vi "DAISY_HIGHSPEED_slow_control_2_16.vi"() -> ()   [LabVIEW 2018]
uses:
  4623b864-5764-45c6-9cb2-3e18237880ca.vi
  fa57f61f-0bb9-49ac-92eb-fcb40add4dbb.vi
  <vilib>/DAQmx/read.llb/DAQmx Read (Analog 1D DBL NChan 1Samp).vi
  ffb0d1b3-ef19-4e2e-b36e-7277177ef4b3.vi
  9a1acc8a-69db-4048-9e4c-bb07d66d2422.vi
  <vilib>/DAQmx/create/channels.llb/DAQmx Create Channel (AI-Voltage-Basic).vi
  <vilib>/DAQmx/create/channels.llb/DAQmx Create Channel (AI-Current-Basic).vi
  <vilib>/DAQmx/create/channels.llb/DAQmx Create Channel (AI-Temperature-RTD).vi
  <vilib>/DAQmx/miscellaneous.llb/DAQmx Fill In Error Info.vi
  <vilib>/Utility/file.llb/Read Delimited Spreadsheet (string).vi
  <instrlib>/Lake Shore 335/Lake Shore 335.lvlib
  <instrlib>/CAEN PSM/CAEN PSM.lvlib
  <resource>/objmgr/daqmx.rc
panel:
  out "Heater":dbl
  out "Coldhead":dbl
  out "Cycle number":i32
  out "Alarm state":bool
  out "Timestamp last \nmeasured (UPS)":timestamp
  out "Auto-clear":bool
  in  "Auto-clear data?":bool
  in  "Clear data":bool
  in  "Clear data every N cycles":dbl=1000000.0
  in  "N samples":i32=30
  out "Average Flow (SLPM)":dbl caption="Flow (SLPM)"
  out "CAEN Ch. Names":string[](array[string])
  in  "Cycles to execute":dbl=5.0 format="%#_13g"
  out "Detector Pressure":dbl
  in  "N samples":i32=20
  in  "Allows tabs on \nfront panel":T1(tab)
  in  "Anode ch.":enum16{"1", "2", "3", "4"}(ring)=enum."3"
  in  "CAEN unit selector":enum16{"CAEN 1", "CAEN 2"}(ring)
  in  "Multipliers":dbl[](array[numeric])=[1.0, 1.0, 1.0, 1.0, 1.0, 1.0, 1.0, 1.0]
  in  "Offsets\nsubtracted":dbl[](array[numeric])=[0.0, 0.0, 0.0, 0.0, 0.0, 0.0, 0.0, 0.0]
  in  "Channel Names (9207, ai8:15)":string[](array[string])=["i0", "i1", "i2", "i3", "i4", "i5", "i6", "i7"] caption="\"Other\""
  in  "Flow meter input:":u16(ring)=3 items=["v0", "v1", "v2", "v3", "v4", "v5", "v6", "v7"]
  in  "Detector pressure input:":u16(ring) items=["v0", "v1", "v2", "v3", "v4", "v5", "v6", "v7"]
  in  "Channel Names (9207, ai0:7)":string[](array[string])=["v0", "v1", "v2", "v3", "v4", "v5", "v6", "v7"] caption="\"Other\""
  in  "Multipliers":dbl[](array[numeric])=[1.0, 1.0, 1.0, 1.0, 1.0, 1.0, 1.0, 1.0]
  in  "Offsets\nsubtracted":dbl[](array[numeric])=[0.0, 0.0, 0.0, 0.0, 0.0, 0.0, 0.0, 0.0]
  in  "Voltage channels":tag[](array[tag])=["9207/ai0", "9207/ai1", "9207/ai2", "9207/ai3", "9207/ai4", "9207/ai5", "9207/ai6", "9207/ai7"]
  in  "COM-port CAEN":refnum<visa-resource-name>
  in  "ID Query":bool
  in  "COM-port LakeShore":refnum<visa-resource-name>
  in  "PID settings":cluster{"P":dbl, "I":dbl, "D":dbl}={"P"=50.0, "I"=20.0, "D"=120.0}
  in  "Current channels":tag[](array[tag])=["9207/ai8", "9207/ai9", "9207/ai10", "9207/ai11", "9207/ai12", "9207/ai13", "9207/ai14", "9207/ai15"]
  in  "Channel Names (CAEN)":string[](array[string])=["PMT 1", "PMT 2", "Anode", "Cathode", "Top gate", "Bottom gate", "Other 1", "Other 2"]
  in  "RTD Type":i32(ring)=10071 items=["Pt3750"=12481, "Pt3851"=10071, "Pt3911"=12482, "Pt3916"=10069, "Pt3920"=10053, "Pt3928"=12483, "Custom"=10137]
  in  "Module 1 channels (slot 1)":tag[](array[tag])=["cDAQ2Mod2/ai0", "cDAQ2Mod2/ai1", "cDAQ2Mod2/ai2", "cDAQ2Mod2/ai3", "cDAQ2Mod2/ai4", "cDAQ2Mod2/ai5", "cDAQ2Mod2/ai6", "cDAQ2Mod2/ai7"]
  in  "Resistance Configuration":i32(ring)=3 items=["3-Wire"=3, "4-Wire"=4]
  in  "R (T = 0°C):":dbl=100.0 format="%_4g"
  in  "B":dbl
  in  "A":dbl
  in  "C":dbl
  in  "Module 2 channels (slot 2)":tag[](array[tag])=["cDAQ2Mod3/ai0", "cDAQ2Mod3/ai1", "cDAQ2Mod3/ai2", "cDAQ2Mod3/ai3", "cDAQ2Mod3/ai4", "cDAQ2Mod3/ai5", "cDAQ2Mod3/ai6", "cDAQ2Mod3/ai7"]
  in  "Shut off heater \nif Alarm is active":bool=TRUE
  in  "Re-save headers":bool
  in  "Resistance Configuration":i32(ring)=3 items=["3-Wire"=3, "4-Wire"=4]
  in  "Module 3 channels":tag[](array[tag])
  in  "RTD Type":i32(ring)=12481 items=["Pt3750"=12481, "Pt3851"=10071, "Pt3911"=12482, "Pt3916"=10069, "Pt3920"=10053, "Pt3928"=12483, "Custom"=10137]
  in  "R (T = 0°C)":dbl=1000.0 format="%0.1f"
  in  "Ignore Initialization Errors":bool=TRUE caption="Ignore init. errors?"
  out "Started up?":bool
  out "heater":i32
  in  "Kill all channels":bool
  in  "Scale.Range:Minimum 8":dbl
  in  "Scale.Range:Maximum 8":dbl=4000.0
  in  "Scale.Range:Minimum 7":dbl
  in  "Scale.Range:Maximum 7":dbl=4000.0
  in  "Scale.Range:Minimum 6":dbl=-3000.0
  in  "Scale.Range:Maximum 6":dbl
  in  "Scale.Range:Minimum 5":dbl
  in  "Scale.Range:Maximum 5":dbl=3000.0
  in  "Scale.Range:Minimum 4":dbl=-5000.0
  in  "Scale.Range:Maximum 4":dbl
  in  "Scale.Range:Maximum 3":dbl=4000.0
  in  "Scale.Range:Minimum 3":dbl
  in  "Scale.Range:Maximum 2":dbl=1000.0
  in  "Scale.Range:Minimum 2":dbl
  out "CAEN 1.1":dbl(knob) scale=0.0..1000.0
  out "CAEN 1.1":string
  in  "Scale.Range:Maximum":dbl=1000.0
  in  "Scale.Range:Minimum":dbl
  out "CAEN 2.3 2":string
  out "CAEN 2.2 2":string
  out "Channel Names":string[](array[string])
  out "CAEN 2.3":dbl(knob) scale=0.0..4000.0
  out "CAEN 2.2":dbl(knob) scale=0.0..4000.0
  out "CAEN 2.1":string
  out "CAEN 2.0":string
  out "CAEN 1.3":string
  out "CAEN 1.2":string
  out "CAEN 1.0":string
  out "Channel Names":string[](array[string])
  in  "Set to zero (ramp down)":bool
  out "CAEN 2.1":dbl(knob) scale=0.0..-3000.0
  out "CAEN 2.0":dbl(knob) scale=0.0..3000.0
  in  "Apply Voltage":bool
  in  "VSet (V)":dbl[](array[numeric])
  in  "IMax (uA)":dbl[](array[numeric])
  in  "VMax (V)":dbl[](array[numeric])
  out "CAEN 1.3":dbl(knob) scale=0.0..-5000.0
  out "CAEN 1.2":dbl(knob) scale=0.0..4000.0
  out "CAEN 1.0":dbl(knob) scale=0.0..1000.0
  out "Vmon (V)":dbl[](array[numeric])
  out "IMon (uA)":dbl[](array[numeric])
  in  "Reset anode\nperiodically?":bool
  in  "Kill every Y minutes":i32=10
  in  "Keep off for X seconds":i32=10
  out "?":bool
  out "Killed":bool
  out "Restarted":bool
  out "Anode timers":timestamp[](array[timestamp])
  out "Seconds until \nanode autokill":dbl format="%.2g"
  out "Seconds until \nanode reset":dbl format="%.2g"
  in  "Temperature channel selector":u16(ring) items=["0"=0, "1"=1, "2"=2, "3"=3, "4"=4, "5"=5, "6"=6, "7"=7, "Average"=666]
  out "Heater power (%)":cluster{timestamp[], dbl[]}[](graph)
  out "Flow (SLPM)":cluster{timestamp[], dbl[]}[](graph)
  out "9207 (ai 0:7, Volts)":cluster{timestamp[], dbl[]}[](graph)
  out "Phase Diagram":cluster{"X":dbl, "Y":dbl}[](graph)
  out "Setup Temperature (9216 0:15, °C)":cluster{timestamp[], dbl[]}[](graph)
  out "LakeShore readings":dbl[](array[numeric])
  out "Low Temperature (9226 0:7 and LakeShore A;B, °C)":cluster{timestamp[], dbl[]}[](graph)
  in  "Reset?":bool
  out "Integrated Flow (SL)":dbl
  in  "Pause?":bool
  in  "Setpoint (°C)":dbl=-100.0 format="%.1f"
  in  "Heater range":u16(ring) items=["Off", "Low (On)", "Medium", "High"]
  in  "\"Sound\" alarm":bool
  in  "Sound alarm\nFrequency (Hz)":dbl=1260.0
  in  "Send status email now":bool
  out "Email error":i32
  out "source":string
  in  "Number of Bonus lines":i32=1
  out "Names (optional)":string[](array[string])
  in  "Send daily email?":bool=TRUE
  in  "Phone numbers":string[](array[string])
  out "Alarm (or test) message":string
  in  "Alarm\nMaster switch":bool
  in  "Repeat Alarm SMS\nevery N minutes":dbl=15.0
  in  "Test alarm":bool
  out "Warning":bool
  in  "UPS":bool
  in  "UPS Voltage \nLower Threshold":dbl=220.0
  out "NI mod 2&3 status":bool
  in  "NI mod 2&3":bool
  in  "NI mod 1":bool
  in  "CAEN 2":bool
  in  "CAEN 1":bool
  in  "LakeShore":bool
  out "Det. P. warning":bool
  out "Boolean 6":bool
  out "Boolean 5":bool
  out "Boolean 4":bool
  out "Boolean 3":bool
  out "Boolean 2":bool
  out "Boolean":bool
  in  "T 6":bool
  in  "T 5":bool
  in  "T 4":bool
  in  "T 3":bool
  in  "T 2":bool
  in  "T 1":bool
  in  "Detector Pressure":bool
  in  "Overpressure threshold":dbl
  in  "Underpressure threshold":dbl
  out "Comm. status":bool
  in  "High Temp threshold":dbl format="%#_13g"
  in  "Low Temp threshold":dbl format="%#_13g"
  out "LakeShore status":bool
  out "NI mod1 (P) status":bool
  out "CAEN 1 status":bool
  out "CAEN 2 status":bool
  out "Initialization status":bool
  out "Minimum input voltage measured":dbl
  out "Alarm active 2":bool
  out "SMS error":string
  out "Status email preview":string
  in  "Send status email at time:":string="14:00"
  in  "Email Addresses":string[](array[string])
  in  "return address":string="xamsups@gmail.com"
  out "NI 9226":errorcluster
  in  "HV Channel status":string="Click the button to request the latest High Voltage channel status.\nView another channel with the arrows, or typing 0 through 3."
  out "CAEN 1":T2(array[cluster])
  out "CAEN 2":T2(array[cluster])
  in  "Query HV status":bool
  in  "LabVIEW error code":string="Google this"
  in  "String 7":string="A checkmark means \"No error\" and false. A red X means an error occurred"
  out "\"status\"":bool
  in  "\"source\"":string="This may show two things: the latest executed VI in the task chain, in reverse order, or: which VI produced an error, with a short description. If the error can't easily be resolved, google the code."
  out "NI 9216 x2":errorcluster
  out "CAEN 1":errorcluster
  out "CAEN 2":errorcluster
  out "Lakeshore":errorcluster
  out "NI 9207":errorcluster
  out "Temp A":dbl
  out "Temp B":dbl
  in  "Temperature Channel Selector":u16(ring) items=["0", "1", "2", "3", "4", "5", "6", "7"]
  out "Historical Large Phase Diagram":cluster{dbl[], dbl[]}[](graph)
  out "Large Phase Diagram":cluster{"X":dbl, "Y":dbl}[](graph)
  in  "Temperature Channel Selector":u16(ring) items=["0"=0, "1"=1, "2"=2, "3"=3, "4"=4, "5"=5, "6"=6, "7"=7, "Average"=666]
  out "PT1000 data":dbl[](array[numeric]) format="%0.2f"
  out "9207 (V; A) Converted":dbl[](array[numeric])
  out "9216 #1 (°C)":dbl[](array[numeric])
  out "9216 #2 (°C)":dbl[](array[numeric])
  out "Raw readouts (V, mA)":dbl[](array[numeric]) format="%0.2f"
  out "Det.P input #":i32
  out "Flow input #":i32
  out "PT100 data":dbl[](array[numeric]) format="%0.2f"
  out "9207 (ai 8:15, Amperes)":cluster{timestamp[], dbl[]}[](graph)
  in  "Kill voltage":bool
  in  "stop":bool
  out "Voltages":dbl[](array[numeric])
  out "TOBA appended":dbl[][](array[numeric])
  out "Time until next cycle":dbl format="%.3g"
  in  "Time per cycle (s)":i32=2 caption="Time Target (s)"
  # "<- Proof of concept for New/Old T + New P"
  # "Remove ^this^ array, just for testing and takes up lots of resources"
  # "Moving averages"
  # "CAEN settings"
  # "NI 9216 Temperature settings"
  # "NI 9207 Voltage settings"
  # "NI 9207 Current settings"
  # "If RTD type is custom,\nspecify the Callendar-\nVan Dusen parameters"
  # "Anode connected to:"
  # "Channel:"
  # "Lakeshore settings"
  # "NI 9226 Temperature settings"
  # "Miscellaneous"
  # "Gain (P) (XX.X)"
  # "Reset (I) (XX.X)"
  # "Rate (D) (X.X%)"
  # "Data"
  # "Scale:"
  # "to"
  # "to"
  # "Scale:"
  # "Time of last reset"
  # "Time of last reactivation"
  # "to"
  # "Scale:"
  # "to"
  # "Scale:"
  # "Settings"
  # "Scale:"
  # "to"
  # "Scale:"
  # "to"
  # "Scale:"
  # "to"
  # "to"
  # "Scale:"
  # "Alarm indicators and arms"
  # "Detector Thresholds"
  # "Daily status email"
  # "SMS and sound alarm"
  # "Alarm conditions"
  # "Temperature channels:"
  # "Uninterruptable Power Supply"
  # "Task information"
  # "High Voltage channel status"
  # "Error info example"
  # "Channel"
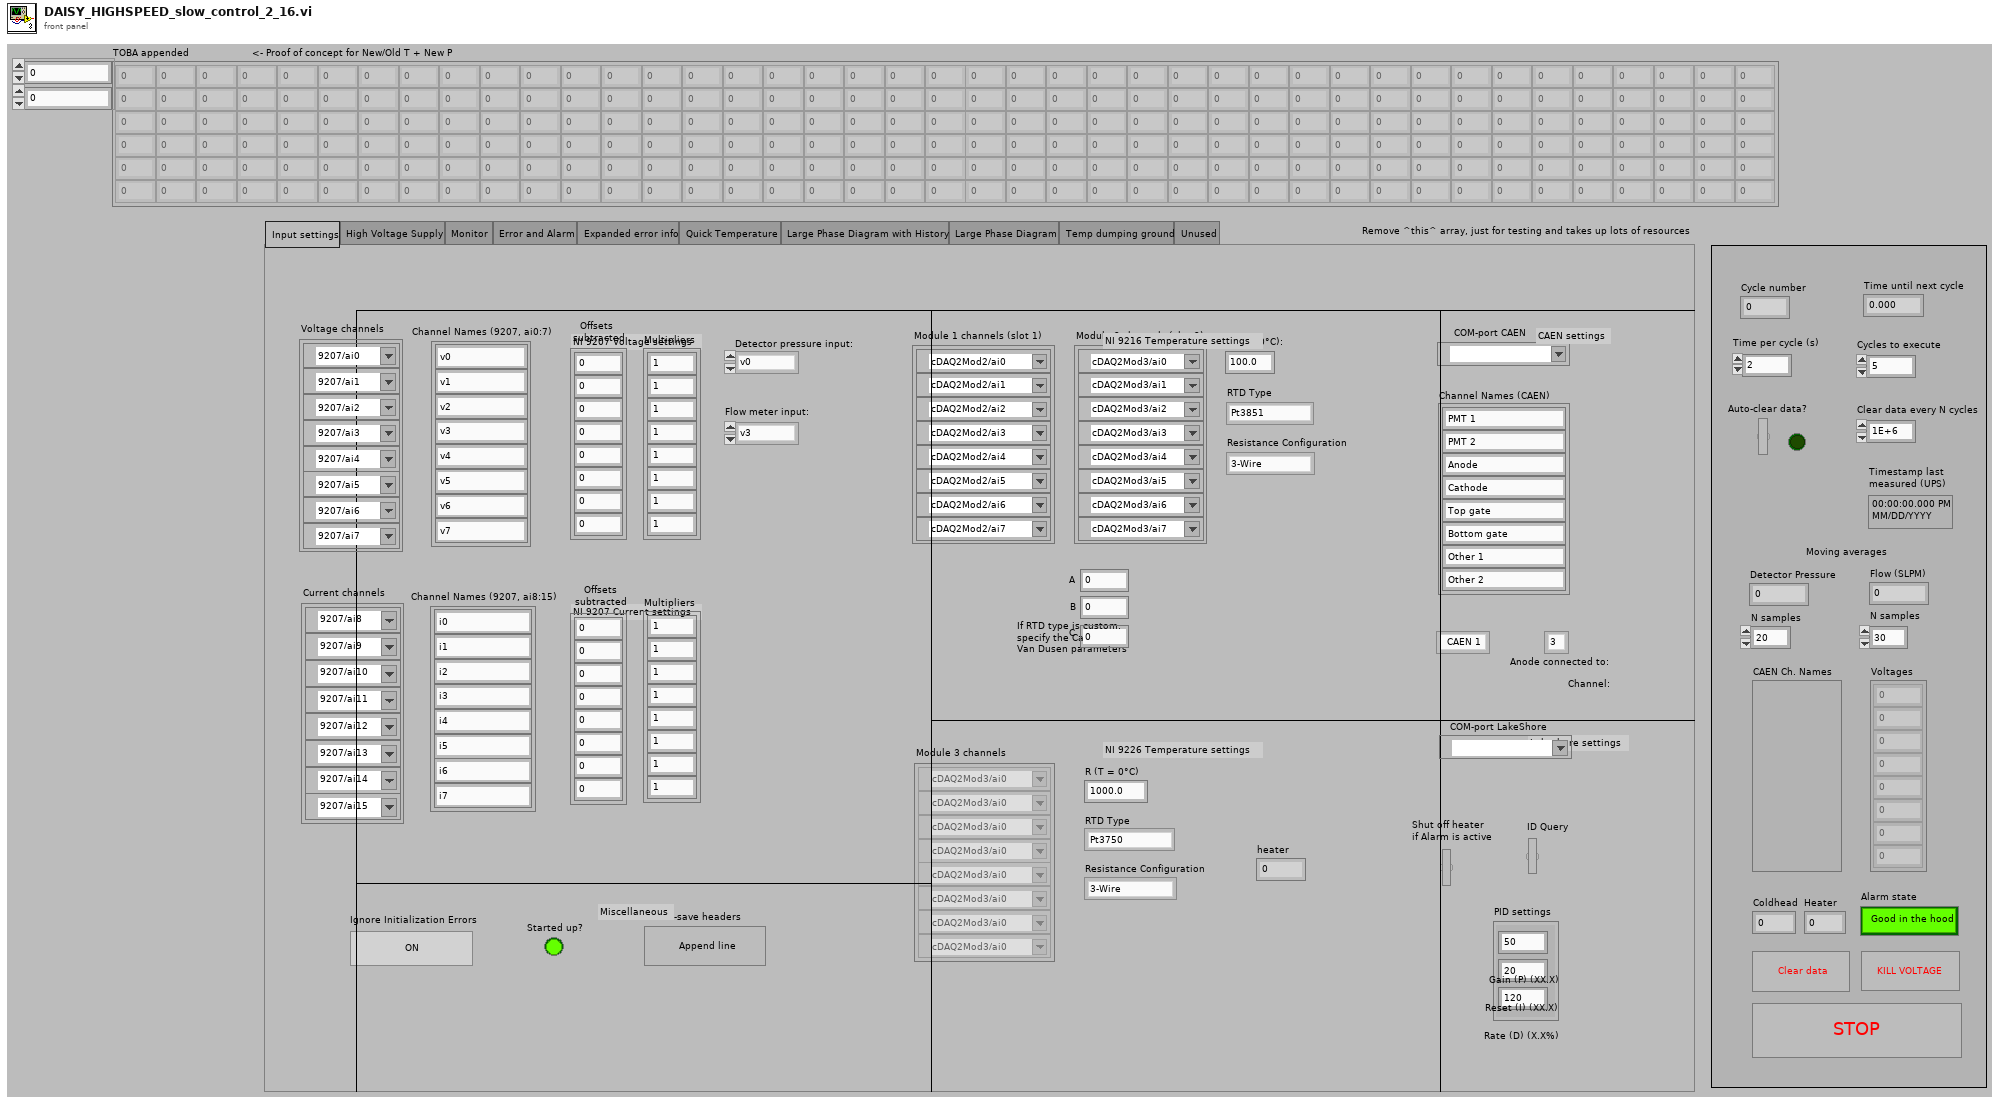
[diagram p1: front panel]
types:
  T1 = enum32{"Input settings", "High Voltage Supply", "Monitor", "Error and Alarm", "Expanded error info", "Quick Temperature", "Large Phase Diagram with History", "Large Phase Diagram", "Temp dumping ground", "Unused"}
  T2 = cluster{"ON":bool, "RUP":bool, "RDW":bool, "OVC":bool, "OVV":bool, "UNV":bool, "MAXV":bool, "TRIP":bool, "OVP":bool, "OVT":bool, "DIS":bool, "KILL":bool, "ILK":bool, "NOCAL":bool}[]
  T3 = cluster{"Baud Rate":u32, "Parity":u16, "Data Bits":u16, "Stop Bits":u16, "Flow Control":u16}
  T4 = typedef "CAEN PSM.lvlib/BoardHandle.ctl" = cluster{"VISA resource name":refnum<visa-resource-name>, "Board address":u8, "NChannels":u8}
  T5 = cluster{"task out":refnum<k21>, "error out":errorcluster}
  T6 = cluster{"VISA resource name out":refnum<visa-resource-name>, "error out":errorcluster}
  T7 = cluster{"VISA resource name":refnum<visa-resource-name>, "Board address":u8, "NChannels":u8}[]
  T8 = cluster{"VISA resource name":refnum<visa-resource-name>, "Board address":u8, "NChannels":u8}
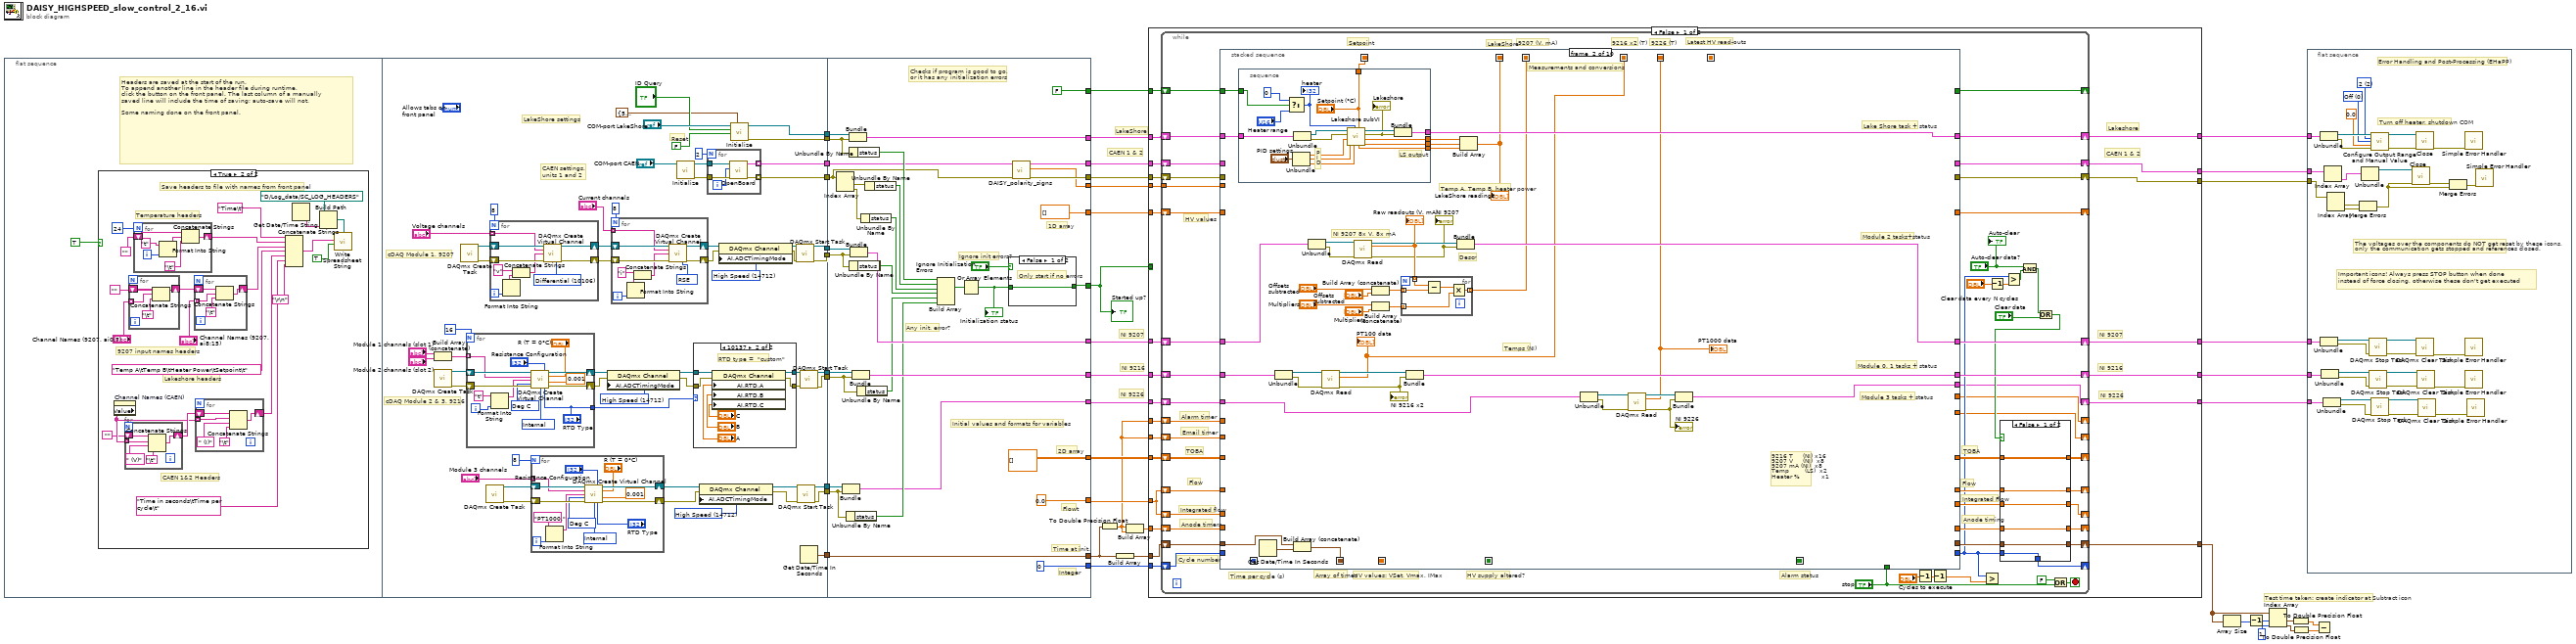
[diagram p0: block diagram]
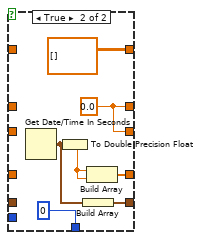
[diagram p2: hidden frame]
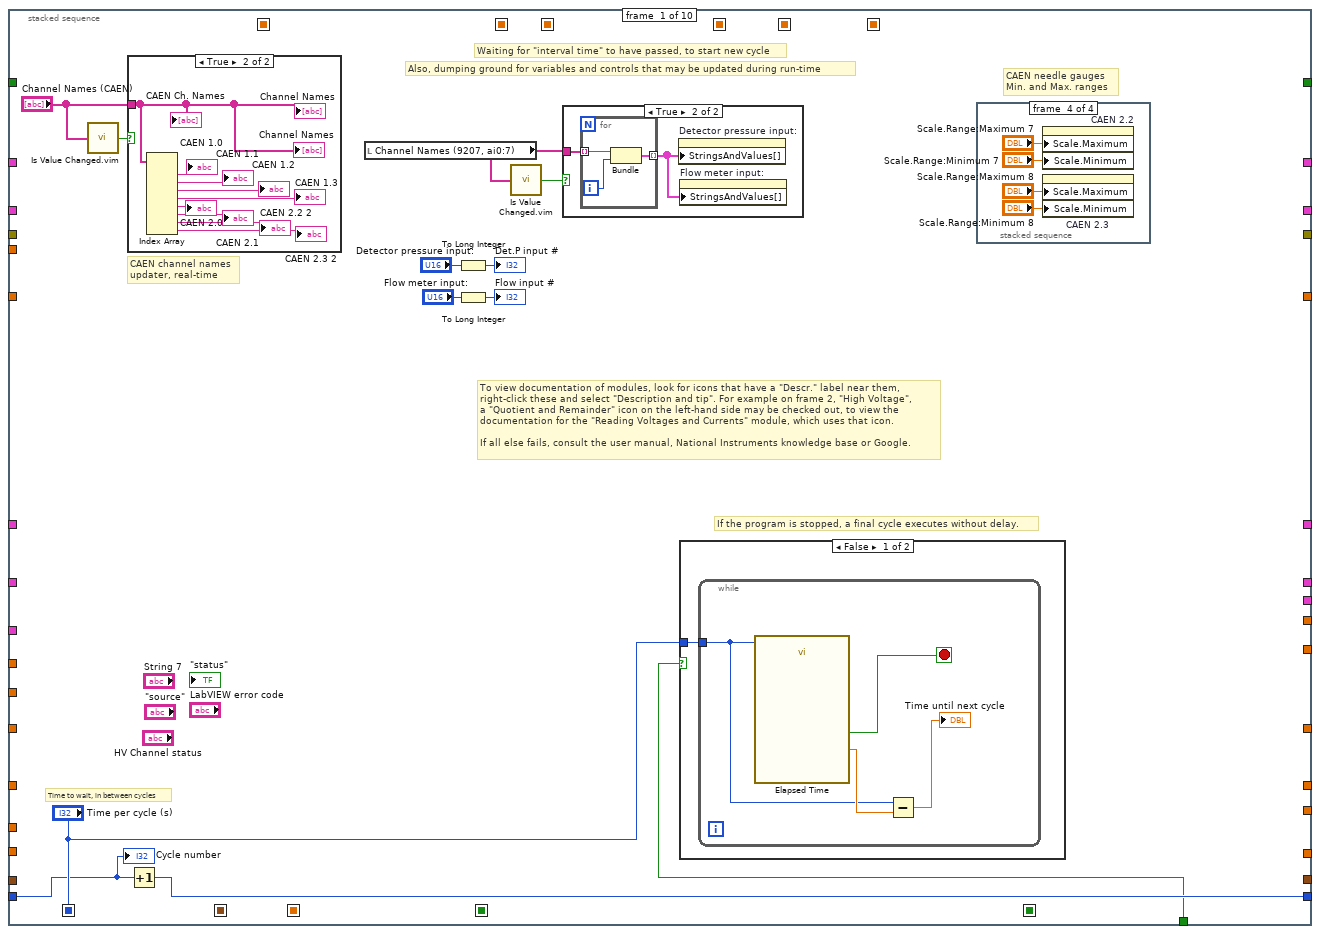
[diagram p3: hidden frame]
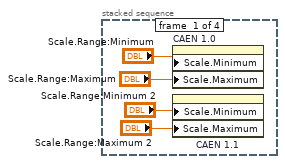
[diagram p6: hidden frame]
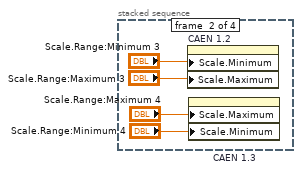
[diagram p7: hidden frame]
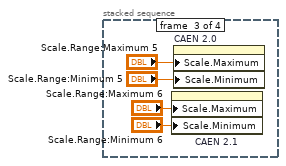
[diagram p8: hidden frame]
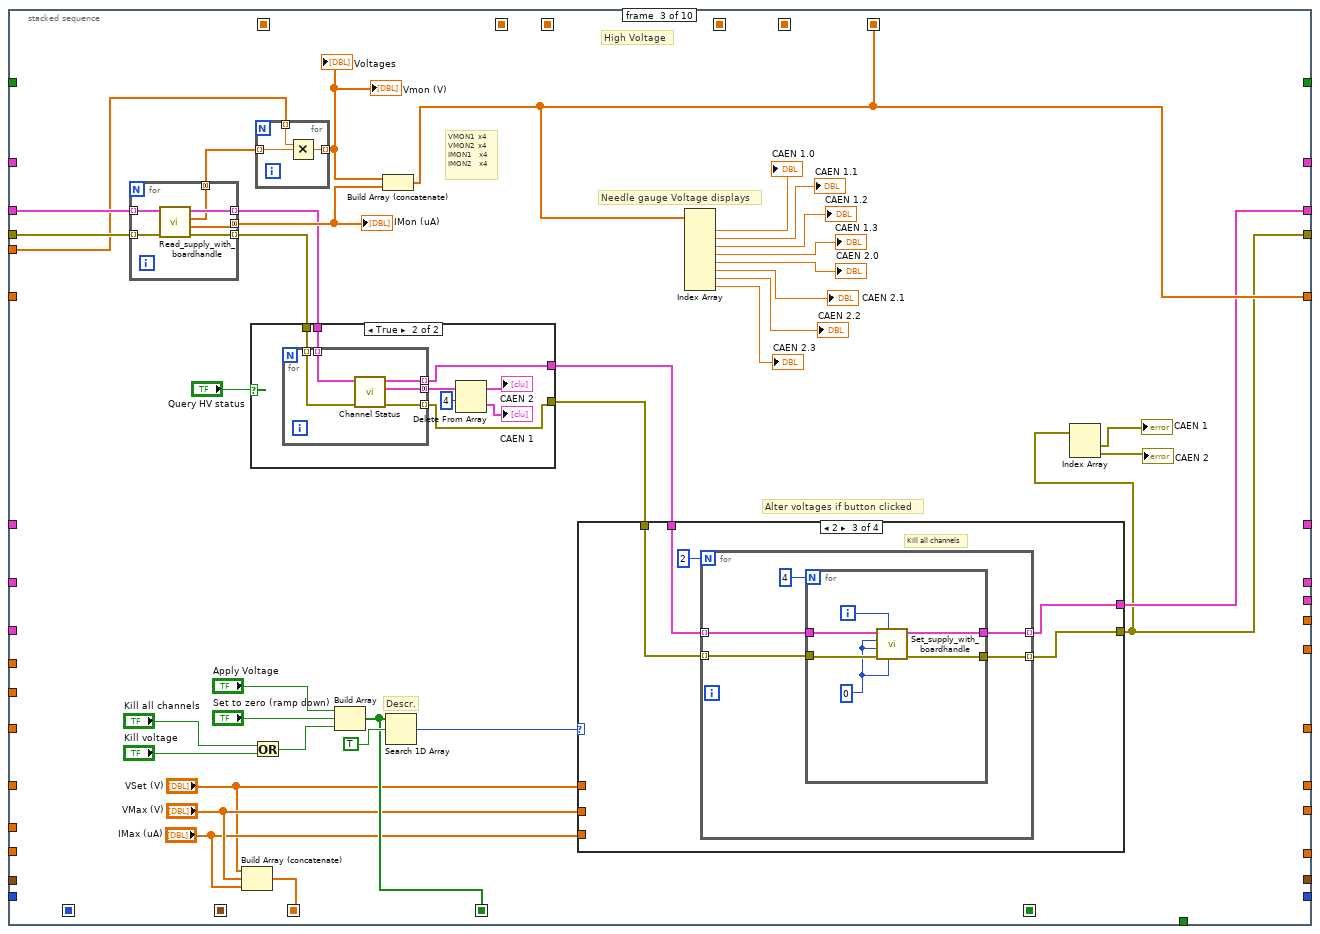
[diagram p10: hidden frame]
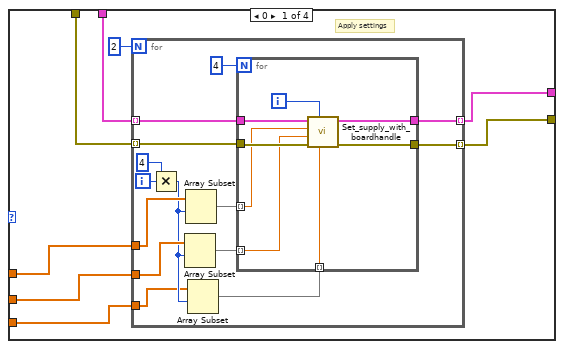
[diagram p11: hidden frame]
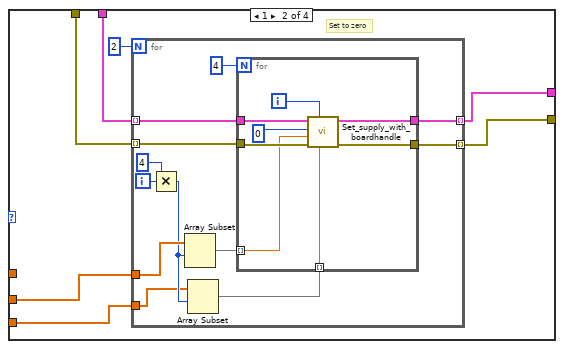
[diagram p12: hidden frame]
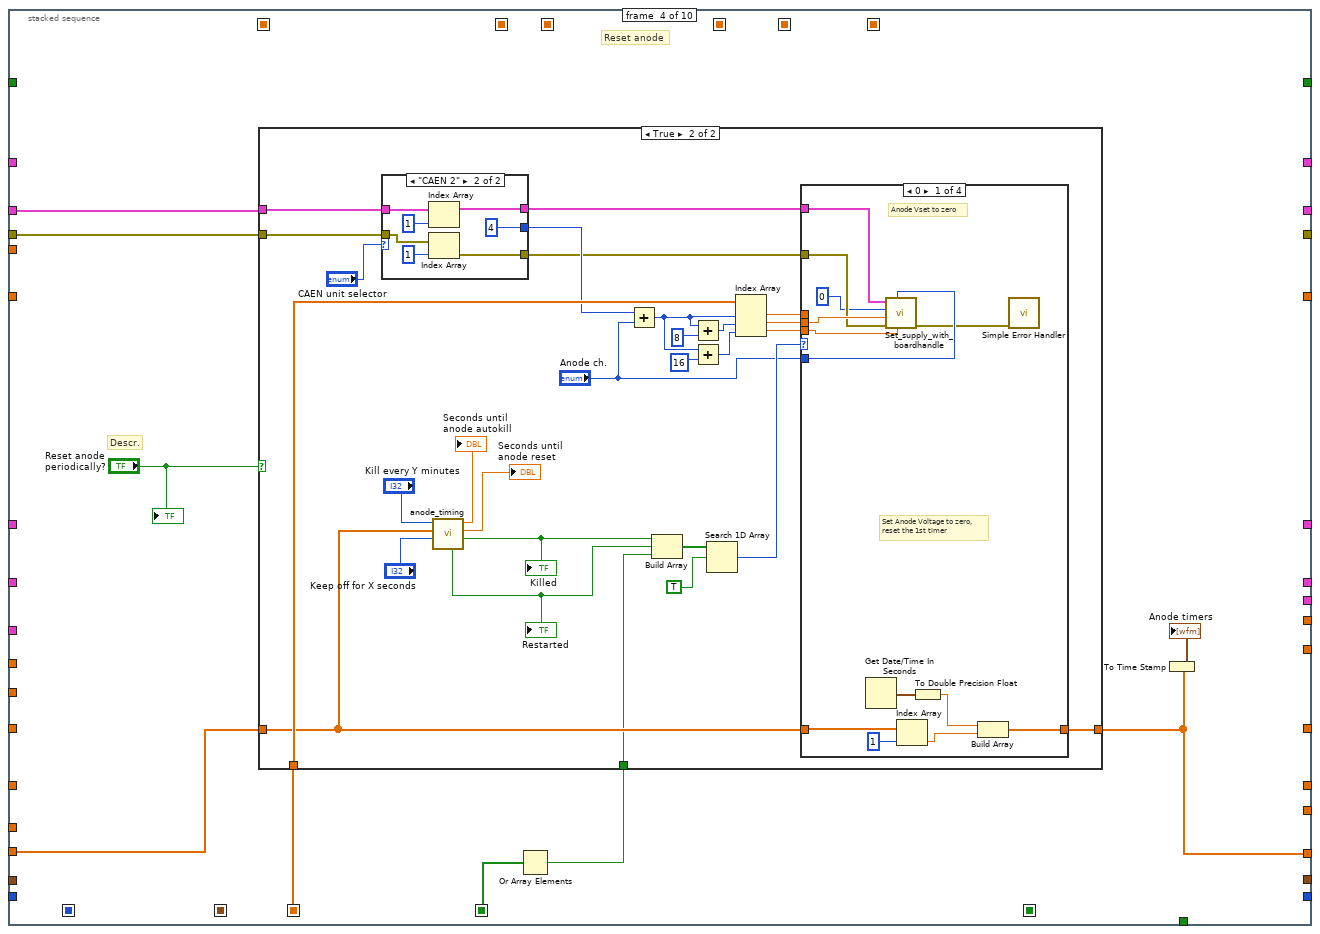
[diagram p15: hidden frame]
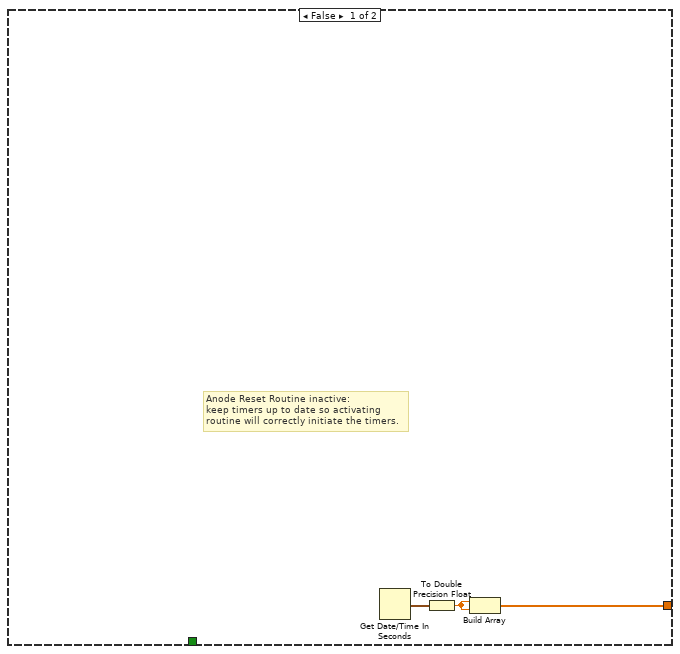
[diagram p16: hidden frame]
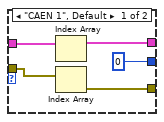
[diagram p17: hidden frame]
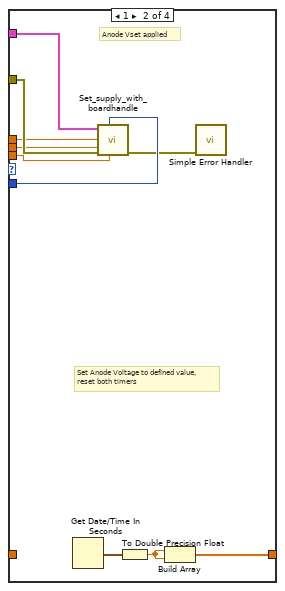
[diagram p18: hidden frame]
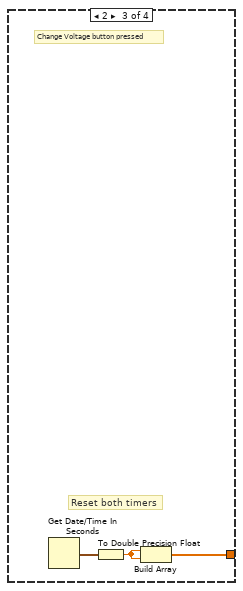
[diagram p19: hidden frame]
diagram:
  # "NI 9226"
  # "NI 9216"
  # "Test time taken: create indicator at Subtract icon"
  # "NI 9207"
  # "CAEN 1 & 2"
  # "LakeShore"
  n1 = flat-sequence {
    tunnel: [w140] -> w42
    tunnel: [w139] -> w41
    tunnel: [w136] -> w40
    tunnel: [w127] -> w39
    tunnel: [w135] -> w35
    tunnel: [w128] -> w21
    tunnel: [w122] -> w14
    tunnel: [w121] -> w13
    tunnel: [w110] -> w9
    tunnel: [w109] -> w8
    tunnel: [w106] -> w4
    tunnel: w42 -> [w237]
    tunnel: w41 -> [w236]
    tunnel: w40 -> [w208]
    tunnel: w39 -> [w229]
    tunnel: [w238] -> w27
    tunnel: [0.0] -> w26
    tunnel: [dbl[] []] -> w38
    tunnel: [dbl[][] []] -> w15
    tunnel: [0] -> w37
    tunnel: [w235] -> w36
    tunnel: [w234] -> w25
    tunnel: w35 -> [w234]
    tunnel: [FALSE] -> w22
    tunnel: w21 -> [w230]
    tunnel: [w228] -> w20
    tunnel: w14 -> [w221]
    tunnel: w13 -> [w220]
    tunnel: [w219] -> w12
    tunnel: w9 -> [w216]
    tunnel: w8 -> [w215]
    tunnel: [w213] -> w7
    tunnel: [w206] -> w5
    tunnel: w4 -> [w210]
    tunnel: [w209] -> w3
    tunnel: [w207] -> w2
    frame #0 {
      # "Headers are saved at the start of the run.\nTo append another line in the header file during runtime,\nclick the button on the front panel. The last column of a manually\nsaved line will include the time of saving; auto-save will not.\n\nSome naming done on the front panel."
      n2 = case shown="True" TRUE {
        frame False {
        }
        frame True {
          # "CAEN 1&2 Headers"
          # "Lakeshore headers"
          # "9207 input names headers"
          # "Temperature headers"
          # "Save headers to file with names from front panel"
          n3 = property on="Channel Names (CAEN)" class="Arr (strict)"() -> ("Value"=w49:string[])  [unwired: 2 in, 2 out]
          n4 = for {
            tunnel: w49 -> [w73] mode=indexing
            shift-right: [w71] -> w50
            shift-left: "" -> [w70]
            n5 = Concatenate Strings(w70, w73, " (V)", "\t") -> (w71:string)
          }
          n6 = for {
            shift-right: [w81] -> w53
            shift-left: "" -> [w82]
            tunnel: "Channel Names (9207, ai0:7)" -> [w79] mode=indexing
            n7 = Concatenate Strings(w82, w79, "\t") -> (w81:string)
          }
          n8 = for {
            N: 24 -> [_]
            shift-right: [w83] -> w56
            shift-left: "" -> [w84]
            i -> [w88]
            n9 = Format Into String(initial string="t", w88) -> (resulting string=w86:string)  [unwired: 2 in, 1 out]
            n10 = Concatenate Strings(w84, w86, "\t") -> (w83:string)
          }
          n11 = for {
            shift-right: [w76] -> w52
            shift-left: w53 -> [w78]
            tunnel: "Channel Names (9207, ai8:15)" -> [w75] mode=indexing
            n12 = Concatenate Strings(w78, w75, "\t") -> (w76:string)
          }
          n13 = for {
            shift-right: [w66] -> w48
            shift-left: w50 -> [w67]
            tunnel: w49 -> [w65] mode=indexing
            n14 = Concatenate Strings(w67, w65, " (I)", "\t") -> (w66:string)
          }
          n15 = Concatenate Strings("Time\t", w56, w52, "Temp A\tTemp B\tHeater Power\tSetpoint\t", w48, "Time in seconds\tTime per cycle\t", "\r\n") -> (w55:string)
          n16 = Get Date/Time String() -> (date string=w59:string)  [unwired: 3 in, 1 out]
          n17 = Build Path(base path=path "D:/Log_data/SC_LOG_HEADERS" ("file path (dialog if empty)"), name or relative path=w59) -> (appended path=w60:path)
          n18 = call <vilib>:"Write Spreadsheet String.vi"("append to file? (new file:F)"=TRUE, "spreadsheet string"=w55, "file path (dialog if empty)"=w60) -> ()  [unwired: 7 in, 2 out]
        }
      }
    }
    frame #1 {
      w89 = 14712 items=["Automatic"=16097, "High Resolution"=10195, "High Speed"=14712, "Best 50 Hz Rejection"=14713, "Best 60 Hz Rejection"=14714, "Custom"=10137] ("AI.ADCTimingMode")
      w94 = 14712 items=["Automatic"=16097, "High Resolution"=10195, "High Speed"=14712, "Best 50 Hz Rejection"=14713, "Best 60 Hz Rejection"=14714, "Custom"=10137] ("AI.ADCTimingMode")
      w101 = 14712 items=["Automatic"=16097, "High Resolution"=10195, "High Speed"=14712, "Best 50 Hz Rejection"=14713, "Best 60 Hz Rejection"=14714, "Custom"=10137] ("AI.ADCTimingMode")
      # "cDAQ Module 2 & 3, 9216"
      # "cDAQ Module 1, 9207"
      # "CAEN settings,\nunits 1 and 2"
      # "Reset"
      # "LakeShore settings"
      n19 = call <vilib>:"DAQmx Create Task.vi"() -> ("task out"=w107:refnum<k21>, "error out"=w123:errorcluster)  [unwired: 14 in]
      n20 = Build Array (concatenate)("Module 1 channels (slot 1)", "Module 2 channels (slot 2)") -> (w118:tag[])
      n21 = call <vilib>:"DAQmx Create Task.vi"() -> ("task out"=w132:refnum<k21>, "error out"=w131:errorcluster)  [unwired: 14 in]
      n22 = for {
        N: 16 -> [_]
        shift-right: [w182] -> w98
        shift-left: w107 -> [w185]
        shift-right: [w183] -> w96
        shift-left: w123 -> [w184]
        tunnel: w118 -> [w181] mode=indexing
        tunnel: ["RTD Type"] -> w115
        i -> [w179]
        w177 = 10200 items=["Internal"=10200, "External"=10167, "None"=10230] ("Current Excitation Source")
        w176 = 10143 items=["Deg C"=10143, "Deg F"=10144, "Kelvins"=10325, "Deg R"=10145, "From Custom Scale"=10065] ("units")
        n23 = Format Into String(initial string="t", w179) -> (resulting string=w178:string)  [unwired: 2 in, 1 out]
        n24 = call-poly <vilib>:"DAQmx Create Virtual Channel.vi"("task in"=w185, "resistance configuration"="Resistance Configuration", "physical channels"=w181, "r0"="R (T = 0°C):", "name to assign"=w178, "units"=w176, "current excitation value"=0.001, "error in"=w184, "current excitation source"=w177, "rtd type"="RTD Type") -> ("task out"=w182:refnum<k21>, "error out"=w183:errorcluster)  [unwired: 4 in]
      }
      n25 = call <vilib>:"DAQmx Create Task.vi"() -> ("task out"=w113:refnum<k21>, "error out"=w112:errorcluster)  [unwired: 14 in]
      n26 = for {
        N: 8 -> [_]
        shift-right: [w201] -> w104
        shift-left: w132 -> [w200]
        shift-right: [w202] -> w129
        shift-left: w131 -> [w198]
        tunnel: "Voltage channels" -> [w199] mode=indexing
        i -> [w204]
        w196 = 10106 items=["Default"=-1, "RSE"=10083, "NRSE"=10078, "Differential"=10106, "Pseudodifferential"=12529] ("input terminal configuration")
        n27 = Format Into String(w204) -> (resulting string=w203:string)  [unwired: 3 in, 1 out]
        n28 = Concatenate Strings("v" ("string"), w203) -> (w197:string)
        n29 = call-poly <vilib>:"DAQmx Create Virtual Channel.vi"("task in"=w200, "input terminal configuration"=w196, "physical channels"=w199, "name to assign"=w197, "error in"=w198) -> ("task out"=w201:refnum<k21>, "error out"=w202:errorcluster)  [unwired: 9 in]
      }
      n30 = for {
        N: 8 -> [_]
        shift-right: [w160] -> w103
        shift-left: w113 -> [w159]
        shift-right: [w161] -> w102
        shift-left: w112 -> [w162]
        tunnel: "Module 3 channels" -> [w157] mode=indexing
        i -> [w155]
        w151 = 10200 items=["Internal"=10200, "External"=10167, "None"=10230] ("current excitation source")
        w153 = 10143 items=["Deg C"=10143, "Deg F"=10144, "Kelvins"=10325, "Deg R"=10145, "From Custom Scale"=10065] ("units")
        n31 = Format Into String(initial string="PT1000.", w155) -> (resulting string=w154:string)  [unwired: 2 in, 1 out]
        n32 = call-poly <vilib>:"DAQmx Create Virtual Channel.vi"("task in"=w159, "resistance configuration"="Resistance Configuration", "physical channels"=w157, "r0"="R (T = 0°C)", "name to assign"=w154, "units"=w153, "current excitation value"=0.001, "error in"=w162, "current excitation source"=w151, "rtd type"="RTD Type") -> ("task out"=w160:refnum<k21>, "error out"=w161:errorcluster)  [unwired: 4 in]
      }
      n33 = property class="DAQmx Channel"(reference=w98, error in=w96, "AI.ADCTimingMode"=w94) -> (reference out=w97:refnum<k21>, error out=w95:errorcluster)
      n34 = for {
        N: 8 -> [_]
        shift-right: [w187] -> w93
        shift-left: w104 -> [w194]
        shift-right: [w186] -> w90
        shift-left: w129 -> [w193]
        tunnel: "Current channels" -> [w192] mode=indexing
        i -> [w191]
        w195 = 10083 items=["default"=-1, "RSE"=10083, "NRSE"=10078, "Differential"=10106, "Pseudodifferential"=12529] ("input terminal configuration")
        n35 = Format Into String(w191) -> (resulting string=w189:string)  [unwired: 3 in, 1 out]
        n36 = Concatenate Strings("i", w189) -> (w188:string)
        n37 = call-poly <vilib>:"DAQmx Create Virtual Channel.vi"("task in"=w194, "input terminal configuration"=w195, "physical channels"=w192, "name to assign"=w188, "error in"=w193) -> ("task out"=w187:refnum<k21>, "error out"=w186:errorcluster)  [unwired: 9 in]
      }
      n38 = call <instrlib>:"Initialize.vi"("VISA resource name"="COM-port CAEN") -> ("error out"=w137:errorcluster, "VISA resource name out"=w133:refnum<visa-resource-name>)  [unwired: 9 in]
      n39 = case shown="10137" w115 {
        tunnel: w97 -> [w164 w168]
        tunnel: w95 -> [w163 w167]
        tunnel: [w164 w166] -> w117
        tunnel: [w163 w165] -> w116
        frame 0, Default {
          # "Don't need to specify the A, B, C\nvalues if RTD type is not \"custom\""
        }
        frame 10137 {
          # "RTD type =  \"custom\""
          n40 = property class="DAQmx Channel"(reference=w168, error in=w167, "AI.RTD.A"="A", "AI.RTD.B"="B", "AI.RTD.C"="C") -> (reference out=w166:refnum<k21>, error out=w165:errorcluster)
        }
      }
      n41 = property class="DAQmx Channel"(reference=w103, error in=w102, "AI.ADCTimingMode"=w101) -> (reference out=w100:refnum<k21>, error out=w99:errorcluster)
      n42 = for {
        N: 2 -> [_]
        tunnel: w133 -> [w146]
        tunnel: [w144] -> w106 mode=indexing
        tunnel: w137 -> [w148]
        tunnel: [w147] -> w136 mode=indexing
        i -> [w145]
        n43 = call <instrlib>:"OpenBoard.vi"("error in (no error)"=w148, "Board Address"=w145, "VISA resource name"=w146) -> ("error out"=w147:errorcluster, "BoardHandle"=w144:T4)  [unwired: 7 in]
      }
      n44 = property class="DAQmx Channel"(reference=w93, error in=w90, "AI.ADCTimingMode"=w89) -> (reference out=w92:refnum<k21>, error out=w91:errorcluster)
      n45 = call <instrlib>:"Initialize.vi"("Serial Configuration"=T3 {"Baud Rate"=57600, "Parity"=1, "Data Bits"=7, "Stop Bits"=10, "Flow Control"=0}, "Reset (True)"=FALSE ("Reset (LakeShore)"), "ID Query (True)"="ID Query", "VISA resource name"="COM-port LakeShore") -> ("error out"=w139:errorcluster, "VISA resource name out"=w140:refnum<visa-resource-name>)  [unwired: 6 in]
      n46 = call <vilib>:"DAQmx Start Task.vi"("task/channels in"=w92, "error in"=w91) -> ("task out"=w128:refnum<k21>, "error out"=w127:errorcluster)  [unwired: 12 in]
      n47 = call <vilib>:"DAQmx Start Task.vi"("task/channels in"=w100, "error in"=w99) -> ("task out"=w110:refnum<k21>, "error out"=w109:errorcluster)  [unwired: 12 in]
      n48 = call <vilib>:"DAQmx Start Task.vi"("task/channels in"=w117, "error in"=w116) -> ("task out"=w122:refnum<k21>, "error out"=w121:errorcluster)  [unwired: 12 in]
      n49 = Get Date/Time In Seconds() -> (seconds since 1Jan1904=w135:timestamp)
    }
    frame #2 {
      # "1D array"
      # "Initial values and formats for variables"
      # "Time at init."
      # "Integer"
      # "2D array"
      # "Flowt"
      # "Checks if program is good to go,\nor it has any initialization errors"
      # "Ignore init errors?"
      # "Any init. error?"
      n50 = Index Array(array=w208) -> (element #1=w212:errorcluster, element #2=w211:errorcluster)  [unwired: 2 in]
      n51 = Bundle("task out"=w216, "error out"=w215) -> (w213:T5)  [unwired: 1 in]
      n52 = Unbundle By Name(w215) -> ("status"=w214:bool)
      n53 = Unbundle By Name(w236) -> ("status"=w222:bool)
      n54 = Bundle("VISA resource name out"=w237, "error out"=w236) -> (w235:T6)  [unwired: 1 in]
      n55 = Unbundle By Name(w229) -> ("status"=w223:bool)
      n56 = Bundle("task out"=w230, "error out"=w229) -> (w228:T5)  [unwired: 1 in]
      n57 = Bundle("task out"=w221, "error out"=w220) -> (w219:T5)  [unwired: 1 in]
      n58 = Unbundle By Name(w220) -> ("status"=w218:bool)
      n59 = Unbundle By Name(w211) -> ("status"=w233:bool)
      n60 = Unbundle By Name(w212) -> ("status"=w239:bool)
      n61 = Build Array(w222, w239, w223, w233, w218, w214) -> (w240:bool[])
      n62 = Or Array Elements(Boolean array=w240) -> (logical OR=w217:bool)
      "Initialization status" <- w217
      n63 = case shown="False" "Ignore Initialization Errors" {
        tunnel: [w241 FALSE] -> w238
        tunnel: w217 -> [w241 _]
        frame False {
          # "Only start if no errors"
        }
        frame True {
          # "Always start program"
        }
      }
      n64 = call "DAISY_polarity_signs.vi"("Errors in"=w208, "BoardHandles"=w210) -> ("Errors out"=w207:errorcluster[], "Polarity signs"=w206:dbl[], "BoardHandles Out"=w209:T7)  [unwired: 7 in]
    }
  }
  n65 = To Double Precision Float(number=w25) -> (double precision float=w10:dbl)
  n66 = Build Array(w25) -> (w34:timestamp[])
  n67 = Build Array(w10, w10) -> (w24:dbl[])
  n68 = case shown="False" w27 {
    selector: w27 -> [_ w1091]
    tunnel: [_ w1091] -> _
    tunnel: w38 -> [w260 _]
    tunnel: w37 -> [w265 _]
    tunnel: w15 -> [w264 _]
    tunnel: w36 -> [w261 w1089]
    tunnel: w34 -> [w263 _]
    tunnel: [w262 timestamp[] []] -> w30
    tunnel: w26 -> [w256 _]
    tunnel: w24 -> [w259 _]
    tunnel: [w258 w1089] -> w23
    tunnel: w22 -> [w257 _]
    tunnel: w20 -> [w255 w1088]
    tunnel: [w254 w1085] -> w19
    tunnel: [w253 w1088] -> w18
    tunnel: w12 -> [w252 w1087]
    tunnel: [w251 w1087] -> w11
    tunnel: w10 -> [w250 _]
    tunnel: w10 -> [w249 _]
    tunnel: w7 -> [w248 w1086]
    tunnel: [w247 w1086] -> w6
    tunnel: w5 -> [w246 _]
    tunnel: w3 -> [w245 w1085]
    tunnel: w2 -> [w244 w1084]
    tunnel: [w243 w1084] -> w1
    frame False {
      # "NI 9226"
      # "NI 9216"
      # "NI 9207"
      # "CAEN 1 & 2"
      # "Lakeshore"
      n69 = while {
        shift-right: [w281] -> _
        shift-left: w265 -> [w317]
        shift-right: [w294] -> _
        shift-left: w264 -> [w308]
        shift-right: [w286] -> w262
        shift-left: w263 -> [w314]
        shift-right: [w309] -> w254
        shift-left: w245 -> [w303]
        shift-right: [w311] -> _
        shift-left: w260 -> [w313]
        shift-right: [w310] -> w258
        shift-left: w261 -> [w312]
        shift-right: [w290] -> _
        shift-left: w256 -> [w305]
        shift-right: [w292] -> _
        shift-left: w256 -> [w306]
        shift-right: [w288] -> _
        shift-left: w259 -> [w304]
        shift-right: [w276] -> _
        shift-left: w257 -> [w302]
        shift-right: [w300] -> w253
        shift-left: w255 -> [w301]
        shift-right: [w298] -> w251
        shift-left: w252 -> [w299]
        shift-right: [w274] -> _
        shift-left: w250 -> [w275]
        shift-right: [w271] -> _
        shift-left: w249 -> [w272]
        shift-right: [w269] -> w247
        shift-left: w248 -> [w270]
        tunnel: w246 -> [w268]
        shift-right: [w266] -> w243
        shift-left: w244 -> [w267]
        stop <- w315 stop-if-true
        # "9226 (T)"
        # "Email timer"
        # "Alarm timer"
        # "Alarm status"
        # "LakeShore"
        # "9216 x2 (T)"
        # "9207 (V, mA)"
        # "HV supply altered?"
        # "Setpoint"
        # "Anode timing"
        # "Anode timers"
        # "Integrated flow"
        # "Flow"
        # "Flow"
        # "Integrated Flow"
        # "TOBA"
        # "Array of times"
        # "Latest HV read-outs"
        # "Time per cycle (s)"
        # "Cycle number"
        # "HV values: VSet, Vmax, IMax"
        # "HV values"
        # "TOBA"
        n70 = stacked-sequence {
          seq-local: [_ _ w469 _ _ _ _ _ _ _] -> [_ _ _ w581 _ _ _ _ _ _]
          seq-local: ["Time per cycle (s)" _ _ _ _ _ _ _ _ _] -> [_ _ _ _ _ _ w790 _ _ _]
          seq-local: [_ _ w453 _ _ _ _ _ _ _] -> [_ _ _ _ _ _ w788 _ _ _]
          seq-local: [_ w413 _ _ _ _ _ _ _ _] -> [_ _ _ _ w654 w773 _ _ _ _]
          seq-local: [_ _ w465 _ _ _ _ _ _ _] -> [_ _ _ w577 _ _ _ _ _ _]
          seq-local: [_ w407 _ _ _ _ _ _ _ _] -> [_ _ _ _ _ _ w787 _ _ _]
          seq-local: [_ w405 _ _ _ _ _ _ _ _] -> [_ _ _ _ w676 w765 w785 w897 w927 w1013]
          seq-local: [_ w378 _ _ _ _ _ _ _ _] -> [_ _ _ _ w679 w768 w792 _ _ _]
          seq-local: [_ w393 _ _ _ _ _ _ _ _] -> [_ _ _ _ w678 w767 w786 _ _ _]
          seq-local: [_ _ _ _ _ _ _ w857 _ _] -> [_ _ _ _ _ _ _ _ w929 w1014]
          seq-local: [_ w381 _ _ _ _ _ _ _ _] -> [_ _ _ _ w665 _ w784 w855 w923 w996]
          tunnel: [w342 _ _ _ _ _ _ _ _ _] -> w280
          tunnel: "stop" -> [w341 _ _ _ _ _ _ _ _ _]
          tunnel: w317 -> [w331 _ _ _ _ _ _ _ _ _]
          tunnel: w308 -> [_ _ _ _ w708 _ _ _ _ _]
          tunnel: [_ _ _ _ w663 _ _ _ _ _] -> w295
          tunnel: w314 -> [_ w387 _ _ _ _ _ _ _ _]
          tunnel: w303 -> [_ _ w459 w582 _ _ _ _ _ _]
          tunnel: w313 -> [_ _ _ _ _ _ _ _ _ _]
          tunnel: w312 -> [_ w415 _ _ _ _ _ w911 _ _]
          tunnel: [_ w416 _ _ _ _ _ _ _ _] -> w310
          tunnel: [_ _ w453 _ _ _ _ _ _ _] -> w311
          tunnel: [_ _ w446 _ _ _ _ _ _ _] -> w309
          tunnel: [_ _ _ _ w654 _ _ _ _ _] -> w287
          tunnel: w305 -> [_ _ _ _ _ w771 _ _ _ _]
          tunnel: w306 -> [_ _ _ _ _ w772 _ _ _ _]
          tunnel: w304 -> [_ _ _ w583 _ _ _ _ _ _]
          tunnel: [_ _ _ w578 _ _ _ _ _ _] -> w289
          tunnel: w302 -> [_ w409 _ _ _ _ _ _ _ _]
          tunnel: w301 -> [_ w408 _ _ _ _ _ w910 _ _]
          tunnel: [_ w406 _ _ _ _ _ _ _ _] -> w300
          tunnel: [_ _ _ _ _ w770 _ _ _ _] -> w291
          tunnel: [_ _ _ _ _ w769 _ _ _ _] -> w293
          tunnel: w299 -> [_ w392 _ _ _ _ _ w898 _ _]
          tunnel: [_ w388 _ _ _ _ _ _ _ _] -> w298
          tunnel: [_ _ _ _ _ _ _ _ w931 _] -> w276
          tunnel: w275 -> [_ _ _ _ _ _ _ _ w926 _]
          tunnel: [_ _ _ _ _ _ _ _ w924 _] -> w274
          tunnel: w272 -> [_ _ _ _ _ _ _ _ _ w1001]
          tunnel: [_ _ _ _ _ _ _ _ _ w1000] -> w271
          tunnel: w270 -> [_ w386 _ _ _ _ _ _ _ _]
          tunnel: [_ w382 _ _ _ _ _ _ _ _] -> w269
          tunnel: w268 -> [_ _ w456 _ _ _ _ _ _ _]
          tunnel: w267 -> [_ _ w458 w575 _ _ _ w854 _ _]
          tunnel: [_ _ w442 _ _ _ _ _ _ _] -> w266
          frame #0 {
            # "CAEN channel names\nupdater, real-time"
            # "Also, dumping ground for variables and controls that may be updated during run-time"
            # "CAEN needle gauges\nMin. and Max. ranges"
            # "To view documentation of modules, look for icons that have a \"Descr.\" label near them,\nright-click these and select \"Description and tip\". For example on frame 2, \"High Voltage\",\na \"Quotient and Remainder\" icon on the left-hand side may be checked out, to view the\ndocumentation for the \"Reading Voltages and Currents\" module, which uses that icon. \n\nIf all else fails, consult the user manual, National Instruments knowledge base or Google."
            # "Time to wait, in between cycles"
            # "If the program is stopped, a final cycle executes without delay."
            # "Waiting for \"interval time\" to have passed, to start new cycle"
            n71 = call "Is Value Changed.vim"("value"="Channel Names (CAEN)") -> ("changed or first call?"=w334:bool)
            n72 = case shown="True" w334 {
              tunnel: "Channel Names (CAEN)" -> [_ w348]
              frame False {
              }
              frame True {
                n73 = Index Array(array=w348) -> (element #1=→"CAEN 1.0":string, element #2=→"CAEN 1.1":string, element #3=→"CAEN 1.2":string, element #4=→"CAEN 1.3":string, element #5=→"CAEN 2.0":string, element #6=→"CAEN 2.1":string, element #7=→"CAEN 2.2 2":string, element #8=→"CAEN 2.3 2":string)  [unwired: 8 in]
                "CAEN Ch. Names" <- w348
                "Channel Names" <- w348
                "Channel Names" <- w348
              }
            }
            n74 = Increment(x=w331) -> (x+1=w342:i32)
            n75 = local read "Channel Names (9207, ai0:7)"() -> (w332:string[])
            n76 = To Long Integer(number="Detector pressure input:") -> (32bit integer=→"Det.P input #":i32)
            n77 = To Long Integer(number="Flow meter input:") -> (32bit integer=→"Flow input #":i32)
            n78 = call "Is Value Changed.vim"("value"=w332) -> ("changed or first call?"=w333:bool)
            n79 = case shown="True" w333 {
              tunnel: w332 -> [_ w344]
              frame False {
                # ":D"
              }
              frame True {
                n80 = for {
                  tunnel: w344 -> [w347] mode=indexing
                  tunnel: [w345] -> w343 mode=indexing
                  i -> [w346]
                  n81 = Bundle("Or give name if \"Other\""=w347, w346) -> (w345:cluster{"Or give name if \"Other\"":string, i32})  [unwired: 1 in]
                }
                n82 = property on="Detector pressure input:" class="Ring (strict)"("StringsAndValues[]"=w343) -> ()  [unwired: 2 in, 2 out]
                n83 = property on="Flow meter input:" class="Ring (strict)"("StringsAndValues[]"=w343) -> ()  [unwired: 2 in, 2 out]
              }
            }
            n84 = case shown="False" w341 {
              tunnel: "Time per cycle (s)" -> [w373 _]
              frame False {
                n85 = while {
                  tunnel: w373 -> [w375]
                  stop <- w377 stop-if-true
                  n86 = call "Elapsed Time"("Time Target (s)"=w375) -> ("Elapsed Time (s)"=w376:dbl, "Time has Elapsed"=w377:bool)  [unwired: 11 in, 6 out]
                  n87 = Subtract(x=w375, y=w376) -> (x-y=→"Time until next cycle":dbl)
                }
              }
              frame True {
              }
            }
            n88 = stacked-sequence {
              frame #0 {
                n89 = property on="CAEN 1.0" class="Knob (strict)"("Scale.Minimum"="Scale.Range:Minimum", "Scale.Maximum"="Scale.Range:Maximum") -> ()  [unwired: 2 in, 2 out]
                n90 = property on="CAEN 1.1" class="Knob (strict)"("Scale.Minimum"="Scale.Range:Minimum 2", "Scale.Maximum"="Scale.Range:Maximum 2") -> ()  [unwired: 2 in, 2 out]
              }
              frame #1 {
                n91 = property on="CAEN 1.2" class="Knob (strict)"("Scale.Minimum"="Scale.Range:Minimum 3", "Scale.Maximum"="Scale.Range:Maximum 3") -> ()  [unwired: 2 in, 2 out]
                n92 = property on="CAEN 1.3" class="Knob (strict)"("Scale.Maximum"="Scale.Range:Maximum 4", "Scale.Minimum"="Scale.Range:Minimum 4") -> ()  [unwired: 2 in, 2 out]
              }
              frame #2 {
                n93 = property on="CAEN 2.1" class="Knob (strict)"("Scale.Maximum"="Scale.Range:Maximum 6", "Scale.Minimum"="Scale.Range:Minimum 6") -> ()  [unwired: 2 in, 2 out]
                n94 = property on="CAEN 2.0" class="Knob (strict)"("Scale.Maximum"="Scale.Range:Maximum 5", "Scale.Minimum"="Scale.Range:Minimum 5") -> ()  [unwired: 2 in, 2 out]
              }
              frame #3 {
                n95 = property on="CAEN 2.2" class="Knob (strict)"("Scale.Maximum"="Scale.Range:Maximum 7", "Scale.Minimum"="Scale.Range:Minimum 7") -> ()  [unwired: 2 in, 2 out]
                n96 = property on="CAEN 2.3" class="Knob (strict)"("Scale.Maximum"="Scale.Range:Maximum 8", "Scale.Minimum"="Scale.Range:Minimum 8") -> ()  [unwired: 2 in, 2 out]
              }
            }
            "Cycle number" <- w331
          }
          frame #1 {
            # "Module 3 tasks + status"
            # "Module 0, 1 tasks + status"
            # "Lake Shore task + status"
            # "Descr"
            # "NI 9207 8x V, 8x mA"
            # "Module 2 tasks+status"
            # "Temps (NI)"
            # "9216 T     (NI) x16\n9207 V     (NI)  x8\n9207 mA (NI)  x8\nTemp        (LS)  x2\nHeater %           x1"
            # "Temp A, Temp B, heater power"
            # "Measurements and conversions"
            n97 = stacked-sequence {
              tunnel: [w426] -> w416
              tunnel: w415 -> [w425]
              tunnel: [w424] -> w412
              tunnel: [w423] -> w411
              tunnel: [w422] -> w410
              tunnel: w409 -> [w420]
              tunnel: ["Setpoint (°C)"] -> w407
              frame #0 {
                # "LS output"
                # "P\nI\nD"
                n98 = Select(t=0, s=w420, f="Heater range") -> (s? t:f=w417:i32)
                "heater" <- w417
                n99 = Unbundle("PID settings") -> ("P"=w431:dbl, "I"=w430:dbl, "D"=w429:dbl)
                n100 = Unbundle(w425) -> ("VISA resource name out"=w433:refnum<visa-resource-name>, "error out"=w432:errorcluster)
                n101 = call "Lakeshore subVI.vi"("Setpoint"="Setpoint (°C)", "Rate (D) (X.X %)"=w429, "Range"=w417, "Reset (I) (XX.X)"=w430, "Gain (P) (XX.X)"=w431, "error in (no error)"=w432, "VISA resource name"=w433) -> ("Input B"=w423:dbl, "Input A"=w424:dbl, "error out"=w427:errorcluster, "VISA resource name out"=w428:refnum<visa-resource-name>, "Heater 1 (%)"=w422:dbl)
                "Lakeshore" <- w427
                n102 = Bundle("VISA resource name out"=w428, "error out"=w427) -> (w426:T6)  [unwired: 1 in]
              }
            }
            n103 = Get Date/Time In Seconds() -> (seconds since 1Jan1904=w414:timestamp)
            n104 = Unbundle(w392) -> ("task out"=w391:refnum<k21>, "error out"=w390:errorcluster)
            n105 = Build Array (concatenate)(w387, w414) -> (w413:timestamp[])
            n106 = Unbundle(w408) -> ("task out"=w397:refnum<k21>, "error out"=w396:errorcluster)
            n107 = call-poly <vilib>:"DAQmx Read.vi"("task/channels in"=w391, "error in"=w390) -> ("task out"=w380:refnum<k21>, "data"=w378:dbl[], "error out"=w389:errorcluster)  [unwired: 11 in]
            "PT100 data" <- w378
            "NI 9216 x2" <- w389
            n108 = call-poly <vilib>:"DAQmx Read.vi"("task/channels in"=w397, "error in"=w396) -> ("task out"=w395:refnum<k21>, "data"=w404:dbl[], "error out"=w394:errorcluster)  [unwired: 11 in]
            "Raw readouts (V, mA)" <- w404
            "NI 9207" <- w394
            n109 = Build Array (concatenate)("Offsets\nsubtracted", "Offsets\nsubtracted") -> (w398:dbl[])
            n110 = Build Array (concatenate)("Multipliers", "Multipliers") -> (w401:dbl[])
            n111 = for {
              tunnel: w398 -> [w439] mode=indexing
              tunnel: w404 -> [w438] mode=indexing
              tunnel: w401 -> [w436] mode=indexing
              tunnel: [w435] -> w405 mode=indexing
              n112 = Subtract(x=w438, y=w439) -> (x-y=w437:dbl)
              n113 = Multiply(x=w437, y=w436) -> (x*y=w435:dbl)
            }
            n114 = Bundle("task out"=w380, "error out"=w389) -> (w388:T5)  [unwired: 1 in]
            n115 = Bundle("task out"=w395, "error out"=w394) -> (w406:T5)  [unwired: 1 in]
            n116 = Build Array(w412, w411, w410) -> (w393:dbl[])
            "LakeShore readings" <- w393
            n117 = Unbundle(w386) -> ("task out"=w379:refnum<k21>, "error out"=w385:errorcluster)
            n118 = call-poly <vilib>:"DAQmx Read.vi"("task/channels in"=w379, "error in"=w385) -> ("task out"=w384:refnum<k21>, "data"=w381:dbl[], "error out"=w383:errorcluster)  [unwired: 11 in]
            "NI 9226" <- w383
            "PT1000 data" <- w381
            n119 = Bundle("task out"=w384, "error out"=w383) -> (w382:T5)  [unwired: 1 in]
          }
          frame #2 {
            # "Alter voltages if button clicked"
            # "Descr."
            # "VMON1  x4 \nVMON2  x4\nIMON1    x4\nIMON2    x4"
            # "Needle gauge Voltage displays"
            # "High Voltage"
            n120 = for {
              tunnel: w459 -> [w574] mode=indexing
              tunnel: w458 -> [w573] mode=indexing
              tunnel: [w572] -> w451 mode=indexing
              tunnel: [w571] -> w450 mode=indexing
              tunnel: [w570] -> w457 mode=concatenating
              tunnel: [w569] -> w454 mode=concatenating
              n121 = call "Read_supply_with_boardhandle.vi"("error in (no error)"=w573, "BoardHandle"=w574) -> ("error out"=w571:errorcluster, "IMon values (uA)"=w569:dbl[], "VMon values (V)"=w570:dbl[], "BoardHandle out"=w572:T8)  [unwired: 6 in]
            }
            "IMon (uA)" <- w454
            n122 = Build Array (concatenate)("VSet (V)", "VMax (V)", "IMax (uA)") -> (w469:dbl[])
            n123 = case shown="True" "Query HV status" {
              tunnel: w451 -> [w552 w560]
              tunnel: w450 -> [w551 w559]
              tunnel: [w552 w554] -> w448
              tunnel: [w551 w553] -> w447
              frame False {
              }
              frame True {
                n124 = for {
                  tunnel: w560 -> [w565] mode=indexing
                  tunnel: w559 -> [w564] mode=indexing
                  tunnel: [w563] -> w554 mode=indexing
                  tunnel: [w562] -> w553 mode=indexing
                  tunnel: [w561] -> w558 mode=concatenating
                  n125 = call <instrlib>:"Channel Status.vi"("error in (no error)"=w564, "BoardHandle"=w565) -> ("error out"=w562:errorcluster, "Channel Status Array"=w561:T2, "BoardHandle out"=w563:T4)  [unwired: 7 in]
                }
                n126 = Delete From Array(array=w558, length=4) -> (deleted portion=→"CAEN 1":T2, array with subset deleted=→"CAEN 2":T2)  [unwired: 1 in]
              }
            }
            n127 = Or(x="Kill all channels", y="Kill voltage") -> (x .or. y?=w460:bool)
            n128 = for {
              tunnel: w457 -> [w567] mode=indexing
              tunnel: w456 -> [w568] mode=indexing
              tunnel: [w566] -> w455 mode=indexing
              n129 = Multiply(x=w568, y=w567) -> (x*y=w566:dbl)
            }
            "Voltages" <- w455
            "Vmon (V)" <- w455
            n130 = Build Array("Apply Voltage", "Set to zero (ramp down)", w460) -> (w465:bool[])
            n131 = Build Array (concatenate)(w455, w454) -> (w453:dbl[])
            n132 = Search 1D Array(1D array=w465, element=TRUE) -> (index of element=w449:i32)  [unwired: 1 in]
            n133 = case shown="2" w449 {
              tunnel: w448 -> [w482 w511 w536 w550]
              tunnel: w447 -> [w481 w510 w535 w549]
              tunnel: [w477 w507 w534 w550] -> w446
              tunnel: [w476 w506 w533 w549] -> w442
              tunnel: "VSet (V)" -> [w480 _ _ _]
              tunnel: "VMax (V)" -> [w479 w509 _ _]
              tunnel: "IMax (uA)" -> [w478 w508 _ _]
              frame 0 {
                # "Apply settings"
                n134 = for {
                  N: 2 -> [_]
                  tunnel: w482 -> [w496] mode=indexing
                  tunnel: w481 -> [w495] mode=indexing
                  tunnel: w480 -> [w492]
                  tunnel: w479 -> [w490]
                  tunnel: w478 -> [w488]
                  tunnel: [w485] -> w477 mode=indexing
                  tunnel: [w484] -> w476 mode=indexing
                  i -> [w494]
                  n135 = Multiply(x=4, y=w494) -> (x*y=w489:i32)
                  n136 = Array Subset(array=w490, index=w489) -> (w487:dbl[])  [unwired: 1 in]
                  n137 = Array Subset(array=w492, index=w489) -> (w491:dbl[])  [unwired: 1 in]
                  n138 = Array Subset(array=w488, index=w489) -> (w486:dbl[])  [unwired: 1 in]
                  n139 = for {
                    N: 4 -> [_]
                    tunnel: w496 -> [w504]
                    tunnel: w495 -> [w503]
                    tunnel: w491 -> [w502] mode=indexing
                    tunnel: w487 -> [w501] mode=indexing
                    tunnel: w486 -> [w500] mode=indexing
                    tunnel: [w499] -> w485
                    tunnel: [w498] -> w484
                    i -> [w505]
                    n140 = call "Set_supply_with_boardhandle.vi"("Current Limit (0.00 uA)"=w500, "Channel (0)"=w505, "error in (no error)"=w503, "Voltage Max (0.0 V)"=w501, "Voltage Level (0.0 V)"=w502, "BoardHandle"=w504) -> ("error out"=w498:errorcluster, "BoardHandle out"=w499:T8)  [unwired: 4 in]
                  }
                }
              }
              frame 1 {
                # "Set to zero"
                n141 = for {
                  N: 2 -> [_]
                  tunnel: w511 -> [w523] mode=indexing
                  tunnel: w510 -> [w522] mode=indexing
                  tunnel: w509 -> [w519]
                  tunnel: w508 -> [w517]
                  tunnel: [w514] -> w507 mode=indexing
                  tunnel: [w513] -> w506 mode=indexing
                  i -> [w521]
                  n142 = Multiply(x=4, y=w521) -> (x*y=w518:i32)
                  n143 = Array Subset(array=w519, index=w518) -> (w516:dbl[])  [unwired: 1 in]
                  n144 = Array Subset(array=w517, index=w518) -> (w515:dbl[])  [unwired: 1 in]
                  n145 = for {
                    N: 4 -> [_]
                    tunnel: w523 -> [w531]
                    tunnel: w522 -> [w530]
                    tunnel: w516 -> [w529] mode=indexing
                    tunnel: w515 -> [w528] mode=indexing
                    tunnel: [w527] -> w514
                    tunnel: [w526] -> w513
                    i -> [w532]
                    n146 = call "Set_supply_with_boardhandle.vi"("Current Limit (0.00 uA)"=w528, "Channel (0)"=w532, "error in (no error)"=w530, "Voltage Max (0.0 V)"=w529, "Voltage Level (0.0 V)"=0, "BoardHandle"=w531) -> ("error out"=w526:errorcluster, "BoardHandle out"=w527:T8)  [unwired: 4 in]
                  }
                }
              }
              frame 2 {
                # "Kill all channels"
                n147 = for {
                  N: 2 -> [_]
                  tunnel: w536 -> [w541] mode=indexing
                  tunnel: w535 -> [w540] mode=indexing
                  tunnel: [w539] -> w534 mode=indexing
                  tunnel: [w538] -> w533 mode=indexing
                  n148 = for {
                    N: 4 -> [_]
                    tunnel: w541 -> [w547]
                    tunnel: w540 -> [w546]
                    tunnel: [w545] -> w539
                    tunnel: [w544] -> w538
                    i -> [w548]
                    w543 = 0
                    n149 = call "Set_supply_with_boardhandle.vi"("Current Limit (0.00 uA)"=w543, "Channel (0)"=w548, "error in (no error)"=w546, "Voltage Max (0.0 V)"=w543, "Voltage Level (0.0 V)"=w543, "BoardHandle"=w547) -> ("error out"=w544:errorcluster, "BoardHandle out"=w545:T8)  [unwired: 4 in]
                  }
                }
              }
              frame 3, Default {
                # "Do nothing"
              }
            }
            n150 = Index Array(array=w453) -> (element #1=→"CAEN 1.0":dbl, element #2=→"CAEN 1.1":dbl, element #3=→"CAEN 1.2":dbl, element #4=→"CAEN 1.3":dbl, element #5=→"CAEN 2.0":dbl, element #6=→"CAEN 2.1":dbl, element #7=→"CAEN 2.2":dbl, element #8=→"CAEN 2.3":dbl)  [unwired: 8 in]
            n151 = Index Array(array=w442) -> (element #1=→"CAEN 1":errorcluster, element #2=→"CAEN 2":errorcluster)  [unwired: 2 in]
          }
          frame #3 {
            # "Descr."
            # "Reset anode"
            n152 = Or Array Elements(Boolean array=w577) -> (logical OR=w576:bool)
            n153 = case shown="True" "Reset anode\nperiodically?" {
              tunnel: w583 -> [_ w592]
              tunnel: w582 -> [_ w599]
              tunnel: w581 -> [_ w604]
              tunnel: w576 -> [_ w590]
              tunnel: [w584 w591] -> w578
              tunnel: w575 -> [_ w588]
              frame False {
                # "Anode Reset Routine inactive:\nkeep timers up to date so activating\nroutine will correctly initiate the timers."
                n154 = Get Date/Time In Seconds() -> (seconds since 1Jan1904=w586:timestamp)
                n155 = To Double Precision Float(number=w586) -> (double precision float=w585:dbl)
                n156 = Build Array(w585, w585) -> (w584:dbl[])
              }
              frame True {
                n157 = case shown="\"CAEN 2\"" "CAEN unit selector" {
                  tunnel: w599 -> [w619 w625]
                  tunnel: [0 4] -> w597
                  tunnel: [w617 w623] -> w589
                  tunnel: w588 -> [w616 w621]
                  tunnel: [w615 w620] -> w587
                  frame "CAEN 1", Default {
                    n158 = Index Array(array=w619) -> (element=w617:T4)  [unwired: 1 in]
                    n159 = Index Array(array=w616) -> (element=w615:errorcluster)  [unwired: 1 in]
                  }
                  frame "CAEN 2" {
                    n160 = Index Array(array=w625, index=1) -> (element=w623:T4)
                    n161 = Index Array(array=w621, index=1) -> (element=w620:errorcluster)
                  }
                }
                n162 = call "anode_timing.vi"("Keep off for X seconds"="Keep off for X seconds", "Array of timers"=w592, "Kill every Y minutes"="Kill every Y minutes") -> ("Time to kill"=w606:bool, "Time until reset"=→"Seconds until \nanode reset":dbl, "Time until autokill"=→"Seconds until \nanode autokill":dbl, "Time to reset"=w607:bool)  [unwired: 5 in]
                "Killed" <- w606
                "Restarted" <- w607
                n163 = Add(x=w597, y="Anode ch.") -> (x+y=w595:i32)
                n164 = Build Array(w606, w607, w590) -> (w610:bool[])
                n165 = Add(x=w595, y=8) -> (x+y=w600:i32)
                n166 = Add(x=w595, y=16) -> (x+y=w601:i32)
                n167 = Search 1D Array(1D array=w610, element=TRUE) -> (index of element=w609:i32)  [unwired: 1 in]
                n168 = Index Array(array=w604, index #1=w595, index #2=w600, index #3=w601) -> (element #1=w613:dbl, element #2=w611:dbl, element #3=w612:dbl)
                n169 = case shown="0" w609 {
                  tunnel: w613 -> [_ w641 _ _]
                  tunnel: w611 -> [w633 w642 _ _]
                  tunnel: w612 -> [w632 w643 _ _]
                  tunnel: "Anode ch." -> [w629 w644 _ _]
                  tunnel: w592 -> [w635 _ _ w653]
                  tunnel: [w634 w647 w650 w653] -> w591
                  tunnel: w589 -> [w630 w645 _ _]
                  tunnel: w587 -> [w631 w646 _ _]
                  frame 0 {
                    # "Set Anode Voltage to zero,\nreset the 1st timer"
                    # "Anode Vset to zero"
                    n170 = Get Date/Time In Seconds() -> (seconds since 1Jan1904=w638:timestamp)
                    n171 = call "Set_supply_with_boardhandle.vi"("Current Limit (0.00 uA)"=w632, "Channel (0)"=w629, "error in (no error)"=w631, "Voltage Max (0.0 V)"=w633, "Voltage Level (0.0 V)"=0, "BoardHandle"=w630) -> ("error out"=w628:errorcluster)  [unwired: 4 in, 1 out]
                    n172 = Index Array(array=w635, index=1) -> (element=w636:dbl)
                    n173 = To Double Precision Float(number=w638) -> (double precision float=w637:dbl)
                    n174 = Build Array(w637, w636) -> (w634:dbl[])
                    n175 = call <vilib>:"Simple Error Handler.vi"("error in (no error)"=w628) -> ()  [unwired: 4 in, 5 out]
                  }
                  frame 1 {
                    # "Set Anode Voltage to defined value,\nreset both timers"
                    # "Anode Vset applied"
                    n176 = Get Date/Time In Seconds() -> (seconds since 1Jan1904=w649:timestamp)
                    n177 = call "Set_supply_with_boardhandle.vi"("Current Limit (0.00 uA)"=w643, "Channel (0)"=w644, "error in (no error)"=w646, "Voltage Max (0.0 V)"=w642, "Voltage Level (0.0 V)"=w641, "BoardHandle"=w645) -> ("error out"=w640:errorcluster)  [unwired: 4 in, 1 out]
                    n178 = To Double Precision Float(number=w649) -> (double precision float=w648:dbl)
                    n179 = Build Array(w648, w648) -> (w647:dbl[])
                    n180 = call <vilib>:"Simple Error Handler.vi"("error in (no error)"=w640) -> ()  [unwired: 4 in, 5 out]
                  }
                  frame 2 {
                    # "Change Voltage button pressed"
                    # "Reset both timers"
                    n181 = Get Date/Time In Seconds() -> (seconds since 1Jan1904=w652:timestamp)
                    n182 = To Double Precision Float(number=w652) -> (double precision float=w651:dbl)
                    n183 = Build Array(w651, w651) -> (w650:dbl[])
                  }
                  frame 3, Default {
                    # "Timers stay at previous value,\nso difference between those and\ncurrent time keeps incrementing"
                    # "No event"
                  }
                }
              }
            }
            n184 = To Time Stamp(1:w578) -> (0:→"Anode timers":timestamp[])
            "?" <- "Reset anode\nperiodically?"
          }
          frame #4 {
            # "Det. P"
            # "Flow"
            # "Flexibly acquire indices"
            # "Plots 9207 output vs time"
            # "Descr."
            # "Moving averages"
            # "Historic graphs: Phase, 9207 ai, Flow, Heater, Temperature"
            # "Non-historic Temperature + Det. Pressure"
            # "Updated TOBA >>>"
            # "Descr."
            # "Latest Detector Pressure"
            # "Plots individual lists of Temp. vs. t"
            # "Plots and moving averages"
            n185 = Build Array (concatenate)(w679, w665, w676, w678) -> (w707:dbl[])
            n186 = Build Array (concatenate)(w708, w707) -> (w663:dbl[][])
            "TOBA appended" <- w663
            n187 = Array Size(array=w676) -> (size(s)=w675:i32)
            n188 = Array Size(array=w665) -> (size(s)=w677:i32)
            n189 = Array Size(array=w679) -> (size(s)=w666:i32)
            n190 = Add(x=w666, y=w677) -> (x+y=w661:i32)
            n191 = Add(x=w661, y=w675) -> (x+y=w674:i32)
            n192 = local read "Flow input #"() -> (w685:i32)
            n193 = local read "Det.P input #"() -> (w686:i32)
            n194 = Add(x=w674, y=2 ("disabled index (col)")) -> (x+y=w672:i32)
            n195 = Equal?(x=666, y="Temperature channel selector") -> (x = y?=w701:bool)
            n196 = Index Array(array=w663, index (col)=w672) -> (element=w671:dbl[])  [unwired: 1 in]
            n197 = case shown="True" w701 {
              tunnel: w665 -> [w746 w747]
              tunnel: [w745 w748] -> w699
              tunnel: "Temperature channel selector" -> [w744 _]
              frame False {
                n198 = Index Array(array=w746, index=w744) -> (element=w745:dbl)
              }
              frame True {
                n199 = Add Array Elements(numeric array=w747) -> (sum=w749:dbl)
                n200 = Array Size(array=w747) -> (size(s)=w750:i32)
                n201 = Divide(x=w749, y=w750) -> (x/y=w748:dbl)
              }
            }
            n202 = Add(x=w686, y=w661) -> (x+y=w695:i32)
            n203 = Add(x=w661, y=w685) -> (x+y=w693:i32)
            n204 = Bundle(w654, w671) -> (w668:cluster{timestamp[], dbl[]})  [unwired: 1 in]
            n205 = Build Array(w668) -> (→"Heater power (%)":cluster{timestamp[], dbl[]}[])
            n206 = Add(x=w666, y="Temperature Channel Selector") -> (x+y=w669:i32)
            n207 = Index Array(array=w663, index (col) #1=w695, index (col) #2=w693) -> (element #1=w694:dbl[], element #2=w683:dbl[])  [unwired: 2 in]
            n208 = local read "Det.P input #"() -> (w687:i32)
            n209 = Index Array(array=w663, index (col)=w669) -> (element=w698:dbl[])  [unwired: 1 in]
            n210 = for {
              N: 8 -> [_]
              tunnel: w663 -> [w737]
              tunnel: w654 -> [w730]
              tunnel: [w734] -> w691 mode=indexing
              tunnel: [w729] -> w690 mode=indexing
              tunnel: w661 -> [w727]
              i -> [w733]
              n211 = Add(x=w727, y=8) -> (x+y=w726:i32)
              n212 = Add(x=w727, y=w733) -> (x+y=w736:i32)
              n213 = Add(x=w733, y=w726) -> (x+y=w732:i32)
              n214 = Index Array(array=w737, index (col) #1=w736, index (col) #2=w732) -> (element #1=w735:dbl[], element #2=w731:dbl[])  [unwired: 2 in]
              n215 = Bundle(w730, w735) -> (w734:cluster{timestamp[], dbl[]})  [unwired: 1 in]
              n216 = Bundle(w730, w731) -> (w729:cluster{timestamp[], dbl[]})  [unwired: 1 in]
            }
            "9207 (ai 0:7, Volts)" <- w691
            "9207 (ai 8:15, Amperes)" <- w690
            n217 = Bundle(w698, w694) -> (w712:cluster{dbl[], dbl[]})  [unwired: 1 in]
            n218 = Index Array(array=w676, index=w687) -> (element=w713:dbl)
            n219 = call "moving_avg.vi"("N samples"="N samples", "Array"=w694) -> ("Numeric"=→"Detector Pressure":dbl)  [unwired: 9 in]
            n220 = call "moving_avg.vi"("N samples"="N samples", "Array"=w683) -> ("Numeric"=→"Average Flow (SLPM)":dbl)  [unwired: 9 in]
            n221 = Bundle(w654, w683) -> (w710:cluster{timestamp[], dbl[]})  [unwired: 1 in]
            n222 = Build Array(w712) -> (→"Historical Large Phase Diagram":cluster{dbl[], dbl[]}[])
            n223 = Bundle("Waveform"=w699, w713) -> (w717:cluster{"Waveform":dbl, dbl})  [unwired: 1 in]
            n224 = Build Array(w710) -> (→"Flow (SLPM)":cluster{timestamp[], dbl[]}[])
            n225 = Build Array(w717) -> (→"Phase Diagram":cluster{"Waveform":dbl, dbl}[])
            n226 = for {
              N: w666 -> [_]
              tunnel: w654 -> [w762]
              tunnel: [w761] -> w718 mode=indexing
              tunnel: w663 -> [w760]
              i -> [w758]
              n227 = Index Array(array=w760, index (col)=w758) -> (element=w759:dbl[])  [unwired: 1 in]
              n228 = Bundle(w762, w759) -> (w761:cluster{timestamp[], dbl[]})  [unwired: 1 in]
            }
            "Setup Temperature (9216 0:15, °C)" <- w718
            n229 = Increment(x=w661) -> (x+1=w662:i32)
            n230 = Array Size(array=w665) -> (size(s)=w664:i32)
            n231 = Equal?(x=666, y="Temperature Channel Selector") -> (x = y?=w703:bool)
            n232 = Index Array(array=w663, index (col) #1=w661, index (col) #2=w662) -> (element #1=w660:dbl[], element #2=w659:dbl[])  [unwired: 2 in]
            n233 = local read "Channel Names (9207, ai0:7)"() -> (w688:string[])
            n234 = local read "Channel Names (9207, ai8:15)"() -> (w689:string[])
            n235 = case shown="False" w703 {
              tunnel: w665 -> [w753 w754]
              tunnel: [w752 w755] -> w706
              tunnel: "Temperature Channel Selector" -> [w751 _]
              frame False {
                n236 = Index Array(array=w753, index=w751) -> (element=w752:dbl)
              }
              frame True {
                n237 = Add Array Elements(numeric array=w754) -> (sum=w756:dbl)
                n238 = Array Size(array=w754) -> (size(s)=w757:i32)
                n239 = Divide(x=w756, y=w757) -> (x/y=w755:dbl)
              }
            }
            n240 = for {
              N: w664 -> [_]
              tunnel: w654 -> [w725]
              tunnel: [w724] -> w658 mode=indexing
              tunnel: w663 -> [w723]
              tunnel: w666 -> [w719]
              i -> [w720]
              n241 = Add(x=w719, y=w720) -> (x+y=w721:i32)
              n242 = Index Array(array=w723, index (col)=w721) -> (element=w722:dbl[])  [unwired: 1 in]
              n243 = Bundle(w725, w722) -> (w724:cluster{timestamp[], dbl[]})  [unwired: 1 in]
            }
            n244 = Bundle(w654, w660) -> (w657:cluster{timestamp[], dbl[]})  [unwired: 1 in]
            n245 = Bundle(w654, w659) -> (w656:cluster{timestamp[], dbl[]})  [unwired: 1 in]
            n246 = call "Is Value Changed.vim"("value"=w689) -> ("changed or first call?"=w696:bool)
            n247 = call "Is Value Changed.vim"("value"=w688) -> ("changed or first call?"=w697:bool)
            n248 = case shown="True" w696 {
              tunnel: w689 -> [_ w738]
              frame False {
              }
              frame True {
                n249 = for {
                  tunnel: w738 -> [w739] mode=indexing
                  i -> [w740]
                  n250 = property on="9207 (ai 8:15, Amperes)" class="XYGraph (strict)"("Active Plot"=w740, "Plot.Plot Name"=w739) -> ()  [unwired: 2 in, 2 out]
                }
              }
            }
            n251 = case shown="True" w697 {
              tunnel: w688 -> [_ w741]
              frame False {
              }
              frame True {
                n252 = for {
                  tunnel: w741 -> [w742] mode=indexing
                  i -> [w743]
                  n253 = property on="9207 (ai 0:7, Volts)" class="XYGraph (strict)"("Active Plot"=w743, "Plot.Plot Name"=w742) -> ()  [unwired: 2 in, 2 out]
                }
              }
            }
            n254 = Bundle("Waveform"=w706, w713) -> (w715:cluster{"Waveform":dbl, dbl})  [unwired: 1 in]
            n255 = Build Array (concatenate)(w658, w657, w656) -> (→"Low Temperature (9226 0:7 and LakeShore A;B, °C)":cluster{timestamp[], dbl[]}[])
            n256 = Build Array(w715) -> (→"Large Phase Diagram":cluster{"Waveform":dbl, dbl}[])
          }
          frame #5 {
            # "Temp A, Temp B, Heater%"
            # "Temperatures x16\nTo indicators on the physical schematic"
            # "Individual latest 9207 readings.\nIndicators go here. Array is 1x16,\nitems have been converted using\nthe offsets and multipliers"
            # "Displays"
            n257 = local read "Flow input #"() -> (w766:i32)
            n258 = case shown="False" "Reset?" {
              tunnel: [w778 0.0] -> w774
              tunnel: w771 -> [w778 _]
              frame False {
              }
              frame True {
              }
            }
            n259 = Index Array(array=w765) -> ()  [unwired: 16 in, 16 out]
            n260 = Index Array(array=w765, index=w766) -> (element=w769:dbl)
            n261 = call "Average_flow_x_time.vi"("Array of timestamps"=w773, "Previous Flow"=w772, "Latest Flow"=w769) -> ("Volume (SL)"=w775:dbl)  [unwired: 8 in]
            n262 = case shown="False" "Pause?" {
              tunnel: w774 -> [w782 w783]
              tunnel: w775 -> [w781 _]
              tunnel: [w780 w783] -> w770
              frame False {
                n263 = Add(x=w781, y=w782) -> (x+y=w780:dbl)
              }
              frame True {
              }
            }
            "Integrated Flow (SL)" <- w770
            n264 = Index Array(array=w767) -> (element #1=→"Coldhead" →"Temp A":dbl, element #2=→"Heater" →"Temp B":dbl)  [unwired: 3 in, 1 out]
            n265 = Index Array(array=w768) -> ()  [unwired: 16 in, 16 out]
            "9207 (V; A) Converted" <- w765
            "9216 #1 (°C)" <- w768
            "9216 #2 (°C)" <- w768
          }
          frame #6 {
            # "The same order applies to the headers resaved,\nbut with an additional line, stating the date/time"
            # "-----------DATA SAVED----------\nHuman-readable timestamp  ;\nTemperatures (16),  2xNI 9216;\nTemperatures (8),        NI 9226;\nVolts, Amps  (8 x2),     NI 9207;\nTemperature (2),    Lakeshore;\nHeater power (1),  Lakeshore;\nSetpoint (1),           Lakeshore;\nHV readouts (16)          CAEN ;\nCurrent time (s)                ---   ;\nCycle time (s)                    ---   ;"
            # "Saving data"
            n266 = Get Date/Time In Seconds() -> (seconds since 1Jan1904=w806:timestamp)
            n267 = To Double Precision Float(number=w806) -> (double precision float=w789:dbl)
            n268 = Build Array (concatenate)(w792, w784, w785, w786, w787, w788, w789, w790) -> (w805:dbl[])
            n269 = Array Size(array=w792) -> (size(s)=w793:i32)
            n270 = Array Size(array=w784) -> (size(s)=w794:i32)
            n271 = Add(x=w793, y=w794) -> (x+y=w791:i32)
            n272 = Get Date/Time String() -> (date string=w799:string)  [unwired: 3 in, 1 out]
            n273 = case shown="True" "Re-save headers" {
              tunnel: w791 -> [_ w807]
              frame False {
                # "Just sit around and feel pretty"
              }
              frame True {
                w815 = ""
                # "Append line of most recent channel names to header file"
                n274 = local read "Channel Names (CAEN)"() -> (w814:string[])
                n275 = local read "Channel Names (9207, ai0:7)"() -> (w822:string[])
                n276 = for {
                  N: w807 -> [_]
                  shift-right: [w846] -> w818
                  shift-left: "" -> [w847]
                  i -> [w851]
                  n277 = Format Into String(initial string="t", w851) -> (resulting string=w849:string)  [unwired: 2 in, 1 out]
                  n278 = Concatenate Strings(w847, w849, "\t") -> (w846:string)
                }
                n279 = for {
                  shift-right: [w844] -> w820
                  shift-left: w815 -> [w845]
                  tunnel: w822 -> [w842] mode=indexing
                  n280 = Concatenate Strings(w845, w842, "\t") -> (w844:string)
                }
                n281 = local read "Channel Names (9207, ai8:15)"() -> (w821:string[])
                n282 = for {
                  tunnel: w814 -> [w836] mode=indexing
                  shift-right: [w834] -> w809
                  shift-left: w815 -> [w833]
                  n283 = Concatenate Strings(w833, w836, " (V)", "\t") -> (w834:string)
                }
                n284 = for {
                  shift-right: [w840] -> w817
                  shift-left: w820 -> [w841]
                  tunnel: w821 -> [w838] mode=indexing
                  n285 = Concatenate Strings(w841, w838, "\t") -> (w840:string)
                }
                n286 = for {
                  tunnel: w814 -> [w831] mode=indexing
                  shift-right: [w829] -> w813
                  shift-left: w809 -> [w828]
                  n287 = Concatenate Strings(w828, w831, " (I)", "\t") -> (w829:string)
                }
                n288 = Get Date/Time String() -> (date string=w826:string)  [unwired: 3 in, 1 out]
                n289 = Format Date/Time String() -> (date/time string=w808:string)  [unwired: 3 in]
                n290 = Build Path(base path=path "D:/Log_data/SC_LOG_HEADERS", name or relative path=w826) -> (appended path=w825:path)
                n291 = Concatenate Strings("Time\t", w818, w817, "Temp A\tTemp B\tHeater Power\tSetpoint\t", w813, "Time in seconds\tTime per cycle\t", w808, "\r\n") -> (w810:string)
                n292 = call <vilib>:"Write Spreadsheet String.vi"("append to file? (new file:F)"=TRUE, "spreadsheet string"=w810, "file path (dialog if empty)"=w825) -> ()  [unwired: 7 in, 2 out]
              }
            }
            n293 = Build Path(base path=path "D:/Log_data/SC_LOG", name or relative path=w799) -> (appended path=w798:path)
            n294 = Format Date/Time String() -> (date/time string=w803:string)  [unwired: 3 in]
            n295 = Array To Spreadsheet String(array=w805, 3:"%.3f" ("format string")) -> (spreadsheet string=w801:string)  [unwired: 1 in]
            n296 = Concatenate Strings(w803, "\t", w801) -> (w797:string)
            n297 = call <vilib>:"Write Spreadsheet String.vi"("append to file? (new file:F)"=TRUE, "spreadsheet string"=w797, "file path (dialog if empty)"=w798) -> ()  [unwired: 7 in, 2 out]
          }
          frame #7 {
            # "Status is True if ANY (armed)\ncondition is met"
            # "Detector P. Alert"
            # "Uninteruptable\n Power Supply Alert"
            # "Temp. Warning"
            # "Arms"
            # "Comm. Alert"
            # "Temperature Alert"
            # "Alarm conditions (Temp)"
            # "Check Alarms and Warnings"
            n298 = Index Array(array=w854) -> (element #1=w853:errorcluster, element #2=w852:errorcluster)  [unwired: 2 in]
            n299 = Unbundle By Name(w898) -> ("error out.status"=w880:bool)
            "NI mod 2&3 status" <- w880
            n300 = Unbundle By Name(w911) -> ("error out.status"=w909:bool)
            "LakeShore status" <- w909
            n301 = Unbundle By Name(w910) -> ("error out.status"=w906:bool)
            "NI mod1 (P) status" <- w906
            n302 = Unbundle By Name(w852) -> ("status"=w907:bool)
            "CAEN 2 status" <- w907
            n303 = Unbundle By Name(w853) -> ("status"=w908:bool)
            "CAEN 1 status" <- w908
            n304 = Build Array(w909, w908, w907, w906, w880) -> (w881:bool[])
            n305 = Build Array("LakeShore", "CAEN 1", "CAEN 2", "NI mod 2&3", "NI mod 1") -> (w876:bool[])
            n306 = call "check_ups.vi"() -> ("Error: no voltages read"=w860:bool, "Timestamp last measured"=→"Timestamp last \nmeasured (UPS)":timestamp, "Minimum input voltage measured"=w870:dbl)  [unwired: 8 in, 1 out]
            "Minimum input voltage measured" <- w870
            n307 = property on="Det.P input #" class="DigNum (strict)"() -> ("Value"=w896:i32)  [unwired: 2 in, 2 out]
            n308 = Or Array Elements(Boolean array=w881) -> (logical OR=→"Comm. status":bool)
            n309 = for {
              tunnel: w881 -> [w914] mode=indexing
              tunnel: w876 -> [w913] mode=indexing
              tunnel: [w912] -> w875 mode=indexing
              n310 = And(x=w914, y=w913) -> (x .and. y?=w912:bool)
            }
            n311 = Index Array(array=w897, index=w896) -> (element=w893:dbl)
            n312 = Less?(x=w870, y="UPS Voltage \nLower Threshold") -> (x < y?=w862:bool)
            n313 = Equal?(x=w870, y=-1.0) -> (x = y?=w861:bool)
            n314 = Less?(x=w893, y="Underpressure threshold") -> (x < y?=w891:bool)
            n315 = Build Array(w862, w861, w860) -> (w859:bool[])
            n316 = Or Array Elements(Boolean array=w875) -> (logical OR=w865:bool)
            n317 = Greater?(x=w893, y="Overpressure threshold") -> (0:w892:bool)
            n318 = Or(x=w892, y=w891) -> (x .or. y?=w890:bool)
            "Det. P. warning" <- w890
            n319 = Or Array Elements(Boolean array=w859) -> (logical OR=w858:bool)
            "Warning" <- w858
            n320 = And(x="UPS", y=w858) -> (x .and. y?=w864:bool)
            n321 = And(x=w890, y="Detector Pressure") -> (x .and. y?=w866:bool)
            n322 = Build Array("T 1", "T 2", "T 3", "T 4", "T 5", "T 6") -> (w856:bool[])
            n323 = for {
              tunnel: w855 -> [w915] mode=indexing
              tunnel: w856 -> [w918] mode=indexing
              tunnel: [w917] -> w867 mode=indexing
              tunnel: [w916] -> w882 mode=indexing
              n324 = Less?(x=w915, y="Low Temp threshold") -> (x < y?=w920:bool)
              n325 = Greater?(x=w915, y="High Temp threshold") -> (0:w919:bool)
              n326 = Or(x=w920, y=w919) -> (x .or. y?=w916:bool)
              n327 = And(x=w918, y=w916) -> (x .and. y?=w917:bool)
            }
            n328 = Index Array(array=w882) -> (element #1=→"Boolean":bool, element #2=→"Boolean 2":bool, element #3=→"Boolean 3":bool, element #4=→"Boolean 4":bool, element #5=→"Boolean 5":bool, element #6=→"Boolean 6":bool)  [unwired: 6 in]
            n329 = Build Array (concatenate)(w867, w866, w865, w864) -> (w863:bool[])
            n330 = Or Array Elements(Boolean array=w863) -> (logical OR=w857:bool)
            "Alarm state" <- w857
          }
          frame #8 {
            # "Testing alarm will not interfere"
            # "Act on alarm"
            n331 = Or(x="Test alarm", y=w929) -> (x .or. y?=w930:bool)
            n332 = case shown="True" w930 {
              tunnel: "Test alarm" -> [_ w937]
              tunnel: w927 -> [_ w945]
              tunnel: w923 -> [_ w944]
              tunnel: w926 -> [w933 w935]
              tunnel: "Alarm\nMaster switch" -> [_ w942]
              tunnel: [w933 w936] -> w924
              frame False {
                # "Timer stays at previous value"
              }
              frame True {
                n333 = Get Date/Time In Seconds() -> (seconds since 1Jan1904=w949:timestamp)
                n334 = case shown="True" "\"Sound\" alarm" {
                  frame False {
                  }
                  frame True {
                    n335 = call <vilib>:"Beep.vi"("use system alert? (T)"=FALSE, "duration (msec)"=u32 1000, "frequency (Hz)"="Sound alarm\nFrequency (Hz)") -> ()  [unwired: 9 in]
                  }
                }
                n336 = To Double Precision Float(number=w949) -> (double precision float=w946:dbl)
                n337 = Multiply(x="Repeat Alarm SMS\nevery N minutes", y=60.0) -> (x*y=w938:dbl)
                n338 = Subtract(x=w946, y=w935) -> (x-y=w941:dbl)
                n339 = Greater?(x=w941, y=w938) -> (0:w943:bool)
                n340 = And(x=w942, y=w943) -> (x .and. y?=w940:bool)
                n341 = Or(x=w937, y=w940) -> (x .or. y?=w939:bool)
                n342 = case shown="True" w939 {
                  tunnel: w937 -> [_ w965]
                  tunnel: w945 -> [_ w973]
                  tunnel: w944 -> [_ w954]
                  tunnel: [w953 w963] -> w936
                  tunnel: w935 -> [w953 w962]
                  frame False {
                    # "Alarm not armed, or defined time has not yet passed"
                  }
                  frame True {
                    # "Average T in Det."
                    n343 = local read "Det.P input #"() -> (w978:i32)
                    n344 = case shown="True" w965 {
                      tunnel: ["Error encountered inXAMS! Status:" "TESTING the XAMS alarm. Status:"] -> w972
                      tunnel: [w982 w985] -> w963
                      tunnel: w962 -> [_ w985]
                      frame False {
                        n345 = Get Date/Time In Seconds() -> (seconds since 1Jan1904=w983:timestamp)
                        n346 = To Double Precision Float(number=w983) -> (double precision float=w982:dbl)
                      }
                      frame True {
                      }
                    }
                    n347 = for {
                      tunnel: w954 -> [w987] mode=indexing
                      tunnel: [w994] -> w957 mode=indexing
                      i -> [w988]
                      n348 = Format Into String(format string="%.0f", w988) -> (resulting string=w992:string)  [unwired: 2 in, 1 out]
                      n349 = Format Into String(format string="%.1f", w987) -> (resulting string=w990:string)  [unwired: 2 in, 1 out]
                      n350 = Concatenate Strings("\n" ("format string"), w992, "     " ("format string"), w990) -> (w994:string)
                    }
                    n351 = Index Array(array=w973, index=w978) -> (element=w974:dbl)
                    n352 = Array Size(array=w954) -> (size(s)=w976:i32)
                    n353 = Add Array Elements(numeric array=w954) -> (sum=w977:dbl)
                    n354 = Format Into String(format string="%.3f", w974) -> (resulting string=w968:string)  [unwired: 2 in, 1 out]
                    n355 = Divide(x=w977, y=w976) -> (x/y=w966:dbl)
                    n356 = Format Date/Time String() -> (date/time string=w970:string)  [unwired: 3 in]
                    n357 = Format Into String(format string="%.2f", w966) -> (resulting string=w955:string)  [unwired: 2 in, 1 out]
                    n358 = Concatenate Strings(w972, "\nDate/time: ", w970, "\nDetector Pressure: ", w968, " bar", "\nDetector Temperatures (°C):", "\nCh:   Temp:" ("format string"), w957, "\nAverage detector temperature: ", w955) -> (w961:string)
                    "Alarm (or test) message" <- w961
                    n359 = for {
                      tunnel: w961 -> [w981]
                      tunnel: "Phone numbers" -> [w980] mode=indexing
                      n360 = call "send_sms.vi"("Message content"=w981, "Phone number"=w980) -> ("standard error"=→"SMS error":string)  [unwired: 8 in, 1 out]
                    }
                  }
                }
              }
            }
            n361 = And(x="Shut off heater \nif Alarm is active", y=w929) -> (x .and. y?=w931:bool)
            "Alarm active 2" <- "Alarm\nMaster switch"
          }
          frame #9 {
            # "Daily e-mail"
            n362 = Get Date/Time In Seconds() -> (seconds since 1Jan1904=w1009:timestamp)
            n363 = To Double Precision Float(number=w1009) -> (double precision float=w1008:dbl)
            n364 = Get Date/Time String(want seconds? (F)=FALSE) -> (time string=w1011:string)  [unwired: 2 in, 1 out]
            n365 = Subtract(x=w1008, y=w1001) -> (x-y=w1007:dbl)
            n366 = Equal?(x=w1011, y="Send status email at time:") -> (x = y?=w1004:bool)
            n367 = Greater?(x=w1007, y=62) -> (0:w1003:bool)
            n368 = Build Array("Send daily email?", w1004, w1003) -> (w1002:bool[])
            n369 = And Array Elements(Boolean array=w1002) -> (logical AND=w998:bool)
            n370 = Or(x="Send status email now", y=w998) -> (x .or. y?=w999:bool)
            n371 = case shown="True" w999 {
              tunnel: w996 -> [_ w1016]
              tunnel: w1014 -> [_ w1033]
              tunnel: w1013 -> [_ w1042]
              tunnel: w1001 -> [w1015 _]
              tunnel: [w1015 w1028] -> w1000
              frame False {
              }
              frame True {
                # "Average T in Det."
                n372 = Not Equal To 0?(x="Number of Bonus lines") -> (x != 0?=w1021:bool)
                n373 = case shown="True" w1021 {
                  tunnel: [w1053 w1056] -> w1022
                  tunnel: "Number of Bonus lines" -> [_ w1059]
                  frame False {
                    n374 = Build Array("\n[Flavor text module inactive]") -> (w1053:string[])
                  }
                  frame True {
                    n375 = Build Path(base path=path "C:/Users/xams/Desktop/New XAMS Slow Control", name or relative path="cool_beans.txt") -> (appended path=w1060:path)
                    n376 = call-poly <vilib>:"Read Delimited Spreadsheet.vi"("file path (dialog if empty)"=w1060) -> ("all rows"=w1063:string[][])  [unwired: 9 in, 5 out]
                    n377 = Array Size(array=w1063) -> (size(s)=w1065:i32[])
                    n378 = Index Array(array=w1065) -> (element=w1064:i32)  [unwired: 1 in]
                    n379 = for {
                      N: w1059 -> [_]
                      tunnel: w1064 -> [w1070]
                      tunnel: w1063 -> [w1069]
                      tunnel: [w1066] -> w1057 mode=indexing
                      n380 = Random Number (0-1)() -> (number: 0 to 1=w1073:dbl)
                      n381 = Multiply(x=w1070, y=w1073) -> (x*y=w1072:dbl)
                      n382 = Round To Nearest(number=w1072) -> (nearest integer value=w1071:dbl)
                      n383 = Index Array(array=w1069, index (row)=w1071) -> (element=w1067:string[])  [unwired: 1 in]
                      n384 = Concatenate Strings("\n", w1067) -> (w1066:string)
                    }
                    n385 = Concatenate Strings("\n\nCool beans of the day: ", w1057) -> (w1055:string)
                    n386 = Build Array(w1055) -> (w1056:string[])
                  }
                }
                n387 = local read "Det.P input #"() -> (w1043:i32)
                n388 = for {
                  tunnel: [w1082] -> w1035 mode=indexing
                  tunnel: w1016 -> [w1074] mode=indexing
                  i -> [w1075]
                  n389 = Format Into String(format string="%.0f", w1075) -> (resulting string=w1079:string)  [unwired: 2 in, 1 out]
                  n390 = Format Into String(format string="%.2f", w1074) -> (resulting string=w1077:string)  [unwired: 2 in, 1 out]
                  n391 = Concatenate Strings("\nCh: " ("format string"), w1079, ", Temp: " ("format string"), w1077, "°C." ("format string")) -> (w1082:string)
                }
                n392 = Array Size(array=w1016) -> (size(s)=w1051:i32)
                n393 = Add Array Elements(numeric array=w1016) -> (sum=w1052:dbl)
                n394 = Index Array(array=w1042, index=w1043) -> (element=w1040:dbl)
                n395 = Divide(x=w1052, y=w1051) -> (x/y=w1049:dbl)
                n396 = Format Into String(format string="%.3f", w1040) -> (resulting string=w1038:string)  [unwired: 2 in, 1 out]
                n397 = Format Into String(format string="%.2f", w1049) -> (resulting string=w1032:string)  [unwired: 2 in, 1 out]
                n398 = Select(t="ACTIVE!!!!!", s=w1033, f="inactive.") -> (s? t:f=w1045:string)
                n399 = Concatenate Strings("Hello, XAMS teammembers.", "\n\nThe alarm is currently ", w1045, "\n\nThe latest detector pressure is: ", w1038, " bar." ("format string"), "\nTemperatures inside the detector are:", w1035, "\nThe average detector temperature is ", w1032, "°C." ("format string"), "\n\nThank you for doing your best today, once again!\nRegards, SC.", w1022) -> (w1027:string)
                "Status email preview" <- w1027
                n400 = call "custom_email_program.vi"("mail server"="smtp.nikhef.nl", "return address"="return address", "message"=w1027, "subject ([No Subject])"="XAMS daily status email.", "Email Adresses"="Email Addresses") -> ("error out"=w1019:errorcluster)  [unwired: 6 in]
                n401 = Unbundle By Name(w1019) -> ("code"=→"Email error":i32, "source"=→"source":string)
                n402 = Get Date/Time In Seconds() -> (seconds since 1Jan1904=w1029:timestamp)
                n403 = To Double Precision Float(number=w1029) -> (double precision float=w1028:dbl)
              }
            }
          }
        }
        n404 = Decrement(x="Cycles to execute") -> (x-1=w297:dbl)
        n405 = Decrement(x=w297) -> (x-1=w296:dbl)
        n406 = Greater?(x=w280, y=w296) -> ()  [unwired: 1 out]
        n407 = Decrement(x="Clear data every N cycles") -> (x-1=w277:dbl)
        n408 = Greater?(x=w280, y=w277) -> (0:w279:bool)
        n409 = And(x="Auto-clear data?", y=w279) -> (x .and. y?=w282:bool)
        n410 = Or(x=w282, y="Clear data") -> (x .or. y?=w284:bool)
        n411 = case shown="False" w284 {
          tunnel: w295 -> [w323 _]
          tunnel: [w323 dbl[][] []] -> w294
          tunnel: w293 -> [w322 _]
          tunnel: [w322 w329] -> w292
          tunnel: w291 -> [w321 _]
          tunnel: [w321 w329] -> w290
          tunnel: w289 -> [w320 _]
          tunnel: [w320 w327] -> w288
          tunnel: w287 -> [w319 _]
          tunnel: [w319 w325] -> w286
          tunnel: w280 -> [w318 _]
          tunnel: [w318 0] -> w281
          frame False {
          }
          frame True {
            w329 = 0.0
            n412 = Get Date/Time In Seconds() -> (seconds since 1Jan1904=w326:timestamp)
            n413 = To Double Precision Float(number=w326) -> (double precision float=w328:dbl)
            n414 = Build Array(w326) -> (w325:timestamp[])
            n415 = Build Array(w328, w328) -> (w327:dbl[])
          }
        }
        n416 = Or(x=FALSE, y="stop") -> (x .or. y?=w315:bool)
        "Auto-clear" <- "Auto-clear data?"
      }
    }
    frame True {
    }
  }
  n417 = Array Size(array=w30) -> (size(s)=w33:i32)
  n418 = Decrement(x=w33) -> (x-1=w32:i32)
  n419 = Index Array(array=w30, index #1=w32, index #2=1 ("index")) -> (element #1=w31:timestamp, element #2=w16:timestamp)
  n420 = To Double Precision Float(number=w31) -> (double precision float=w29:dbl)
  n421 = To Double Precision Float(number=w16) -> (double precision float=w28:dbl)
  n422 = flat-sequence {
    tunnel: w23 -> [w1127]
    tunnel: w19 -> [w1099]
    tunnel: w18 -> [w1117]
    tunnel: w11 -> [w1106]
    tunnel: w6 -> [w1103]
    tunnel: w1 -> [w1097]
    frame #0 {
      w1123 = u16 2 items=["1"=1, "2"=2] ("Heater Output (1:1)")
      w1124 = u16 0 items=["Off", "Low (On)", "Medium", "High"] ("Range (0:Off)")
      # "The voltages over the components do NOT get reset by these icons,\nonly the communication gets stopped and references closed."
      # "Important icons! Always press STOP button when done \ninstead of force closing, otherwise these don't get executed"
      # "Turn off heater, shutdown COM"
      # "Error Handling and Post-Processing (EHaPP)"
      n423 = Unbundle(w1127) -> ("VISA resource name out"=w1126:refnum<visa-resource-name>, "error out"=w1125:errorcluster)
      n424 = Unbundle(w1117) -> ("task out"=w1115:refnum<k21>, "error out"=w1113:errorcluster)
      n425 = Unbundle(w1106) -> ("task out"=w1110:refnum<k21>, "error out"=w1108:errorcluster)
      n426 = Unbundle(w1103) -> ("task out"=w1102:refnum<k21>, "error out"=w1101:errorcluster)
      n427 = Index Array(array=w1099) -> (element=w1098:T4)  [unwired: 1 in]
      n428 = Index Array(array=w1097) -> (element #1=w1095:errorcluster, element #2=w1094:errorcluster)  [unwired: 2 in]
      n429 = Merge Errors(w1095, w1094) -> (w1093:errorcluster)
      n430 = Unbundle(w1098) -> ("VISA resource name"=w1118:refnum<visa-resource-name>)  [unwired: 2 out]
      n431 = call <vilib>:"DAQmx Stop Task.vi"("task/channels in"=w1115, "error in"=w1113) -> ("task out"=w1114:refnum<k21>, "error out"=w1112:errorcluster)  [unwired: 12 in]
      n432 = call <vilib>:"DAQmx Stop Task.vi"("task/channels in"=w1110, "error in"=w1108) -> ("task out"=w1109:refnum<k21>, "error out"=w1107:errorcluster)  [unwired: 12 in]
      n433 = call <vilib>:"DAQmx Stop Task.vi"("task/channels in"=w1102, "error in"=w1101) -> ("task out"=w1100:refnum<k21>, "error out"=w1104:errorcluster)  [unwired: 12 in]
      n434 = call <instrlib>:"Configure Output Range and Manual Value.vi"("VISA resource name"=w1126, "Heater Output (1:1)"=w1123, "Range (0:Off)"=w1124, "Manual Output (0.00 %)"=0.0, "error in (no error)"=w1125) -> ("VISA resource name out"=w1121:refnum<visa-resource-name>, "error out"=w1120:errorcluster)  [unwired: 9 in]
      n435 = call <instrlib>:"Close.vi"("error in (no error)"=w1093, "VISA resource name"=w1118) -> ("error out"=w1096:errorcluster)  [unwired: 9 in]
      n436 = call <instrlib>:"Close.vi"("error in (no error)"=w1120, "VISA resource name"=w1121) -> ("error out"=w1119:errorcluster)  [unwired: 9 in]
      n437 = call <vilib>:"DAQmx Clear Task.vi"("task in"=w1114, "error in"=w1112) -> ("error out"=w1116:errorcluster)  [unwired: 13 in]
      n438 = call <vilib>:"DAQmx Clear Task.vi"("task in"=w1109, "error in"=w1107) -> ("error out"=w1111:errorcluster)  [unwired: 13 in]
      n439 = call <vilib>:"DAQmx Clear Task.vi"("task in"=w1100, "error in"=w1104) -> ("error out"=w1105:errorcluster)  [unwired: 13 in]
      n440 = Merge Errors(w1096, w1093) -> (w1092:errorcluster)
      n441 = call <vilib>:"Simple Error Handler.vi"("error in (no error)"=w1119) -> ()  [unwired: 4 in, 5 out]
      n442 = call <vilib>:"Simple Error Handler.vi"("error in (no error)"=w1116) -> ()  [unwired: 4 in, 5 out]
      n443 = call <vilib>:"Simple Error Handler.vi"("error in (no error)"=w1111) -> ()  [unwired: 4 in, 5 out]
      n444 = call <vilib>:"Simple Error Handler.vi"("error in (no error)"=w1105) -> ()  [unwired: 4 in, 5 out]
      n445 = call <vilib>:"Simple Error Handler.vi"("error in (no error)"=w1092) -> ()  [unwired: 4 in, 5 out]
    }
  }
  n446 = Subtract(x=w29, y=w28) -> ()  [unwired: 1 out]
  "Started up?" <- w27
